vi "Create XML with many configs.vi"() -> ()   [LabVIEW 2020]
panel:
  out "Max payload size":dbl=1336.0
  out "Rx UDP Configuration":string="<?xml version=\"1.0\"?>\n<Board xmlns:xsi=\"http://www.w3.org/2001/XMLSchema-instance\" xmlns:xsd=\"http://www.w3.org/2001/XMLSchema\" BoardId=\"1\">\n  <Port PortId=\"0\">\n    <RxUdpSession VlId=\"60\" VLRange=\"1\" Bag=\"0\" Jitter=\"0\" VLBufSize=\"32768\">\n      <RxCommPort ID=\"Rx1\" DomainID=\"1\" SideID=\"1\" LocationID=\"1\" PartitionID=\"1\" UdpSrcPort=\"1\" UdpDstPort=\"1\" UdpMaxMessageSize=\"512\">\n        <Parameter>\n          <name>Param 0</name> <direction>incoming</direction> <encoding>BNR</encoding> <signed>true</signed> <startBit>0 </startBit> <numberOfBits>64</numberOfBits> <scale>1</scale> <offset>0</offset> <unit>V</unit> <defaultValue>0</defaultValue>\n        </Parameter>\n        <Parameter>\n          <name>Param 1</name> <direction>incoming</direction> <encoding>BNR</encoding> <signed>true</signed> <startBit>64 </startBit> <numberOfBits>64</numberOfBits> <scale>1</scale> <offset>0</offset> <unit>V</unit> <defaultValue>0</defaultValue>\n        </Parameter>\n        <Parameter>\n          <name>Param 2</name> <direction>incoming</direction> <encoding>BNR</encoding> <signed>true</signed> <startBit>128 </startBit> <numberOfBits>64</numberOfBits> <scale>1</scale> <offset>0</offset> <unit>V</unit> <defaultValue>0</defaultValue>\n        </Parameter>\n        <Parameter>\n          <name>Param 3</name> <direction>incoming</direction> <encoding>BNR</encoding> <signed>true</signed> <startBit>192 </startBit> <numberOfBits>64</numberOfBits> <scale>1</scale> <offset>0</offset> <unit>V</unit> <defaultValue>0</defaultValue>\n        </Parameter>\n        <Parameter>\n          <name>Param 4</name> <direction>incoming</direction> <encoding>BNR</encoding> <signed>true</signed> <startBit>256 </startBit> <numberOfBits>64</numberOfBits> <scale>1</scale> <offset>0</offset> <unit>V</unit> <defaultValue>0</defaultValue>\n        </Parameter>\n        <Parameter>\n          <name>Param 5</name> <direction>incoming</direction> <encoding>BNR</encoding> <signed>true</signed> <startBit>320 </startBit> <numberOfBits>64</numberOfBits> <scale>1</scale> <offset>0</offset> <unit>V</unit> <defaultValue>0</defaultValue>\n        </Parameter>\n        <Parameter>\n          <name>Param 6</name> <direction>incoming</direction> <encoding>BNR</encoding> <signed>true</signed> <startBit>384 </startBit> <numberOfBits>64</numberOfBits> <scale>1</scale> <offset>0</offset> <unit>V</unit> <defaultValue>0</defaultValue>\n        </Parameter>\n        <Parameter>\n          <name>Param 7</name> <direction>incoming</direction> <encoding>BNR</encoding> <signed>true</signed> <startBit>448 </startBit> <numberOfBits>64</numberOfBits> <scale>1</scale> <offset>0</offset> <unit>V</unit> <defaultValue>0</defaultValue>\n        </Parameter>\n        <Parameter>\n          <name>Param 8</name> <direction>incoming</direction> <encoding>BNR</encoding> <signed>true</signed> <startBit>512 </startBit> <numberOfBits>64</numberOfBits> <scale>1</scale> <offset>0</offset> <unit>V</unit> <defaultValue>0</defaultValue>\n        </Parameter>\n        <Parameter>\n          <name>Param 9</name> <direction>incoming</direction> <encoding>BNR</encoding> <signed>true</signed> <startBit>576 </startBit> <numberOfBits>64</numberOfBits> <scale>1</scale> <offset>0</offset> <unit>V</unit> <defaultValue>0</defaultValue>\n        </Parameter>\n        <Parameter>\n          <name>Param 10</name> <direction>incoming</direction> <encoding>BNR</encoding> <signed>true</signed> <startBit>640 </startBit> <numberOfBits>64</numberOfBits> <scale>1</scale> <offset>0</offset> <unit>V</unit> <defaultValue>0</defaultValue>\n        </Parameter>\n        <Parameter>\n          <name>Param 11</name> <direction>incoming</direction> <encoding>BNR</encoding> <signed>true</signed> <startBit>704 </startBit> <numberOfBits>64</numberOfBits> <scale>1</scale> <offset>0</offset> <unit>V</unit> <defaultValue>0</defaultValue>\n        </Parameter>\n        <Parameter>\n          <name>Param 12</name> <direction>incoming</direction> <encoding>BNR</encoding> <signed>true</signed> <startBit>768 </startBit> <numberOfBits>64</numberOfBits> <scale>1</scale> <offset>0</offset> <unit>V</unit> <defaultValue>0</defaultValue>\n        </Parameter>\n        <Parameter>\n          <name>Param 13</name> <direction>incoming</direction> <encoding>BNR</encoding> <signed>true</signed> <startBit>832 </startBit> <numberOfBits>64</numberOfBits> <scale>1</scale> <offset>0</offset> <unit>V</unit> <defaultValue>0</defaultValue>\n        </Parameter>\n        <Parameter>\n          <name>Param 14</name> <direction>incoming</direction> <encoding>BNR</encoding> <signed>true</signed> <startBit>896 </startBit> <numberOfBits>64</numberOfBits> <scale>1</scale> <offset>0</offset> <unit>V</unit> <defaultValue>0</defaultValue>\n        </Parameter>\n        <Parameter>\n          <name>Param 15</name> <direction>incoming</direction> <encoding>BNR</encoding> <signed>true</signed> <startBit>960 </startBit> <numberOfBits>64</numberOfBits> <scale>1</scale> <offset>0</offset> <unit>V</unit> <defaultValue>0</defaultValue>\n        </Parameter>\n        <Parameter>\n          <name>Param 16</name> <direction>incoming</direction> <encoding>BNR</encoding> <signed>true</signed> <startBit>1024 </startBit> <numberOfBits>64</numberOfBits> <scale>1</scale> <offset>0</offset> <unit>V</unit> <defaultValue>0</defaultValue>\n        </Parameter>\n        <Parameter>\n          <name>Param 17</name> <direction>incoming</direction> <encoding>BNR</encoding> <signed>true</signed> <startBit>1088 </startBit> <numberOfBits>64</numberOfBits> <scale>1</scale> <offset>0</offset> <unit>V</unit> <defaultValue>0</defaultValue>\n        </Parameter>\n        <Parameter>\n          <name>Param 18</name> <direction>incoming</direction> <encoding>BNR</encoding> <signed>true</signed> <startBit>1152 </startBit> <numberOfBits>64</numberOfBits> <scale>1</scale> <offset>0</offset> <unit>V</unit> <defaultValue>0</defaultValue>\n        </Parameter>\n        <Parameter>\n          <name>Param 19</name> <direction>incoming</direction> <encoding>BNR</encoding> <signed>true</signed> <startBit>1216 </startBit> <numberOfBits>64</numberOfBits> <scale>1</scale> <offset>0</offset> <unit>V</unit> <defaultValue>0</defaultValue>\n        </Parameter>\n        <Parameter>\n          <name>Param 20</name> <direction>incoming</direction> <encoding>BNR</encoding> <signed>true</signed> <startBit>1280 </startBit> <numberOfBits>64</numberOfBits> <scale>1</scale> <offset>0</offset> <unit>V</unit> <defaultValue>0</defaultValue>\n        </Parameter>\n        <Parameter>\n          <name>Param 21</name> <direction>incoming</direction> <encoding>BNR</encoding> <signed>true</signed> <startBit>1344 </startBit> <numberOfBits>64</numberOfBits> <scale>1</scale> <offset>0</offset> <unit>V</unit> <defaultValue>0</defaultValue>\n        </Parameter>\n        <Parameter>\n          <name>Param 22</name> <direction>incoming</direction> <encoding>BNR</encoding> <signed>true</signed> <startBit>1408 </startBit> <numberOfBits>64</numberOfBits> <scale>1</scale> <offset>0</offset> <unit>V</unit> <defaultValue>0</defaultValue>\n        </Parameter>\n        <Parameter>\n          <name>Param 23</name> <direction>incoming</direction> <encoding>BNR</encoding> <signed>true</signed> <startBit>1472 </startBit> <numberOfBits>64</numberOfBits> <scale>1</scale> <offset>0</offset> <unit>V</unit> <defaultValue>0</defaultValue>\n        </Parameter>\n        <Parameter>\n          <name>Param 24</name> <direction>incoming</direction> <encoding>BNR</encoding> <signed>true</signed> <startBit>1536 </startBit> <numberOfBits>64</numberOfBits> <scale>1</scale> <offset>0</offset> <unit>V</unit> <defaultValue>0</defaultValue>\n        </Parameter>\n        <Parameter>\n          <name>Param 25</name> <direction>incoming</direction> <encoding>BNR</encoding> <signed>true</signed> <startBit>1600 </startBit> <numberOfBits>64</numberOfBits> <scale>1</scale> <offset>0</offset> <unit>V</unit> <defaultValue>0</defaultValue>\n        </Parameter>\n        <Parameter>\n          <name>Param 26</name> <direction>incoming</direction> <encoding>BNR</encoding> <signed>true</signed> <startBit>1664 </startBit> <numberOfBits>64</numberOfBits> <scale>1</scale> <offset>0</offset> <unit>V</unit> <defaultValue>0</defaultValue>\n        </Parameter>\n        <Parameter>\n          <name>Param 27</name> <direction>incoming</direction> <encoding>BNR</encoding> <signed>true</signed> <startBit>1728 </startBit> <numberOfBits>64</numberOfBits> <scale>1</scale> <offset>0</offset> <unit>V</unit> <defaultValue>0</defaultValue>\n        </Parameter>\n        <Parameter>\n          <name>Param 28</name> <direction>incoming</direction> <encoding>BNR</encoding> <signed>true</signed> <startBit>1792 </startBit> <numberOfBits>64</numberOfBits> <scale>1</scale> <offset>0</offset> <unit>V</unit> <defaultValue>0</defaultValue>\n        </Parameter>\n        <Parameter>\n          <name>Param 29</name> <direction>incoming</direction> <encoding>BNR</encoding> <signed>true</signed> <startBit>1856 </startBit> <numberOfBits>64</numberOfBits> <scale>1</scale> <offset>0</offset> <unit>V</unit> <defaultValue>0</defaultValue>\n        </Parameter>\n        <Parameter>\n          <name>Param 30</name> <direction>incoming</direction> <encoding>BNR</encoding> <signed>true</signed> <startBit>1920 </startBit> <numberOfBits>64</numberOfBits> <scale>1</scale> <offset>0</offset> <unit>V</unit> <defaultValue>0</defaultValue>\n        </Parameter>\n        <Parameter>\n          <name>Param 31</name> <direction>incoming</direction> <encoding>BNR</encoding> <signed>true</signed> <startBit>1984 </startBit> <numberOfBits>64</numberOfBits> <scale>1</scale> <offset>0</offset> <unit>V</unit> <defaultValue>0</defaultValue>\n        </Parameter>\n        <Parameter>\n          <name>Param 32</name> <direction>incoming</direction> <encoding>BNR</encoding> <signed>true</signed> <startBit>2048 </startBit> <numberOfBits>64</numberOfBits> <scale>1</scale> <offset>0</offset> <unit>V</unit> <defaultValue>0</defaultValue>\n        </Parameter>\n        <Parameter>\n          <name>Param 33</name> <direction>incoming</direction> <encoding>BNR</encoding> <signed>true</signed> <startBit>2112 </startBit> <numberOfBits>64</numberOfBits> <scale>1</scale> <offset>0</offset> <unit>V</unit> <defaultValue>0</defaultValue>\n        </Parameter>\n        <Parameter>\n          <name>Param 34</name> <direction>incoming</direction> <encoding>BNR</encoding> <signed>true</signed> <startBit>2176 </startBit> <numberOfBits>64</numberOfBits> <scale>1</scale> <offset>0</offset> <unit>V</unit> <defaultValue>0</defaultValue>\n        </Parameter>\n        <Parameter>\n          <name>Param 35</name> <direction>incoming</direction> <encoding>BNR</encoding> <signed>true</signed> <startBit>2240 </startBit> <numberOfBits>64</numberOfBits> <scale>1</scale> <offset>0</offset> <unit>V</unit> <defaultValue>0</defaultValue>\n        </Parameter>\n        <Parameter>\n          <name>Param 36</name> <direction>incoming</direction> <encoding>BNR</encoding> <signed>true</signed> <startBit>2304 </startBit> <numberOfBits>64</numberOfBits> <scale>1</scale> <offset>0</offset> <unit>V</unit> <defaultValue>0</defaultValue>\n        </Parameter>\n        <Parameter>\n          <name>Param 37</name> <direction>incoming</direction> <encoding>BNR</encoding> <signed>true</signed> <startBit>2368 </startBit> <numberOfBits>64</numberOfBits> <scale>1</scale> <offset>0</offset> <unit>V</unit> <defaultValue>0</defaultValue>\n        </Parameter>\n        <Parameter>\n          <name>Param 38</name> <direction>incoming</direction> <encoding>BNR</encoding> <signed>true</signed> <startBit>2432 </startBit> <numberOfBits>64</numberOfBits> <scale>1</scale> <offset>0</offset> <unit>V</unit> <defaultValue>0</defaultValue>\n        </Parameter>\n        <Parameter>\n          <name>Param 39</name> <direction>incoming</direction> <encoding>BNR</encoding> <signed>true</signed> <startBit>2496 </startBit> <numberOfBits>64</numberOfBits> <scale>1</scale> <offset>0</offset> <unit>V</unit> <defaultValue>0</defaultValue>\n        </Parameter>\n        <Parameter>\n          <name>Param 40</name> <direction>incoming</direction> <encoding>BNR</encoding> <signed>true</signed> <startBit>2560 </startBit> <numberOfBits>64</numberOfBits> <scale>1</scale> <offset>0</offset> <unit>V</unit> <defaultValue>0</defaultValue>\n        </Parameter>\n        <Parameter>\n          <name>Param 41</name> <direction>incoming</direction> <encoding>BNR</encoding> <signed>true</signed> <startBit>2624 </startBit> <numberOfBits>64</numberOfBits> <scale>1</scale> <offset>0</offset> <unit>V</unit> <defaultValue>0</defaultValue>\n        </Parameter>\n        <Parameter>\n          <name>Param 42</name> <direction>incoming</direction> <encoding>BNR</encoding> <signed>true</signed> <startBit>2688 </startBit> <numberOfBits>64</numberOfBits> <scale>1</scale> <offset>0</offset> <unit>V</unit> <defaultValue>0</defaultValue>\n        </Parameter>\n        <Parameter>\n          <name>Param 43</name> <direction>incoming</direction> <encoding>BNR</encoding> <signed>true</signed> <startBit>2752 </startBit> <numberOfBits>64</numberOfBits> <scale>1</scale> <offset>0</offset> <unit>V</unit> <defaultValue>0</defaultValue>\n        </Parameter>\n        <Parameter>\n          <name>Param 44</name> <direction>incoming</direction> <encoding>BNR</encoding> <signed>true</signed> <startBit>2816 </startBit> <numberOfBits>64</numberOfBits> <scale>1</scale> <offset>0</offset> <unit>V</unit> <defaultValue>0</defaultValue>\n        </Parameter>\n        <Parameter>\n          <name>Param 45</name> <direction>incoming</direction> <encoding>BNR</encoding> <signed>true</signed> <startBit>2880 </startBit> <numberOfBits>64</numberOfBits> <scale>1</scale> <offset>0</offset> <unit>V</unit> <defaultValue>0</defaultValue>\n        </Parameter>\n        <Parameter>\n          <name>Param 46</name> <direction>incoming</direction> <encoding>BNR</encoding> <signed>true</signed> <startBit>2944 </startBit> <numberOfBits>64</numberOfBits> <scale>1</scale> <offset>0</offset> <unit>V</unit> <defaultValue>0</defaultValue>\n        </Parameter>\n        <Parameter>\n          <name>Param 47</name> <direction>incoming</direction> <encoding>BNR</encoding> <signed>true</signed> <startBit>3008 </startBit> <numberOfBits>64</numberOfBits> <scale>1</scale> <offset>0</offset> <unit>V</unit> <defaultValue>0</defaultValue>\n        </Parameter>\n        <Parameter>\n          <name>Param 48</name> <direction>incoming</direction> <encoding>BNR</encoding> <signed>true</signed> <startBit>3072 </startBit> <numberOfBits>64</numberOfBits> <scale>1</scale> <offset>0</offset> <unit>V</unit> <defaultValue>0</defaultValue>\n        </Parameter>\n        <Parameter>\n          <name>Param 49</name> <direction>incoming</direction> <encoding>BNR</encoding> <signed>true</signed> <startBit>3136 </startBit> <numberOfBits>64</numberOfBits> <scale>1</scale> <offset>0</offset> <unit>V</unit> <defaultValue>0</defaultValue>\n        </Parameter>\n        <Parameter>\n          <name>Param 50</name> <direction>incoming</direction> <encoding>BNR</encoding> <signed>true</signed> <startBit>3200 </startBit> <numberOfBits>64</numberOfBits> <scale>1</scale> <offset>0</offset> <unit>V</unit> <defaultValue>0</defaultValue>\n        </Parameter>\n        <Parameter>\n          <name>Param 51</name> <direction>incoming</direction> <encoding>BNR</encoding> <signed>true</signed> <startBit>3264 </startBit> <numberOfBits>64</numberOfBits> <scale>1</scale> <offset>0</offset> <unit>V</unit> <defaultValue>0</defaultValue>\n        </Parameter>\n        <Parameter>\n          <name>Param 52</name> <direction>incoming</direction> <encoding>BNR</encoding> <signed>true</signed> <startBit>3328 </startBit> <numberOfBits>64</numberOfBits> <scale>1</scale> <offset>0</offset> <unit>V</unit> <defaultValue>0</defaultValue>\n        </Parameter>\n        <Parameter>\n          <name>Param 53</name> <direction>incoming</direction> <encoding>BNR</encoding> <signed>true</signed> <startBit>3392 </startBit> <numberOfBits>64</numberOfBits> <scale>1</scale> <offset>0</offset> <unit>V</unit> <defaultValue>0</defaultValue>\n        </Parameter>\n        <Parameter>\n          <name>Param 54</name> <direction>incoming</direction> <encoding>BNR</encoding> <signed>true</signed> <startBit>3456 </startBit> <numberOfBits>64</numberOfBits> <scale>1</scale> <offset>0</offset> <unit>V</unit> <defaultValue>0</defaultValue>\n        </Parameter>\n        <Parameter>\n          <name>Param 55</name> <direction>incoming</direction> <encoding>BNR</encoding> <signed>true</signed> <startBit>3520 </startBit> <numberOfBits>64</numberOfBits> <scale>1</scale> <offset>0</offset> <unit>V</unit> <defaultValue>0</defaultValue>\n        </Parameter>\n        <Parameter>\n          <name>Param 56</name> <direction>incoming</direction> <encoding>BNR</encoding> <signed>true</signed> <startBit>3584 </startBit> <numberOfBits>64</numberOfBits> <scale>1</scale> <offset>0</offset> <unit>V</unit> <defaultValue>0</defaultValue>\n        </Parameter>\n        <Parameter>\n          <name>Param 57</name> <direction>incoming</direction> <encoding>BNR</encoding> <signed>true</signed> <startBit>3648 </startBit> <numberOfBits>64</numberOfBits> <scale>1</scale> <offset>0</offset> <unit>V</unit> <defaultValue>0</defaultValue>\n        </Parameter>\n        <Parameter>\n          <name>Param 58</name> <direction>incoming</direction> <encoding>BNR</encoding> <signed>true</signed> <startBit>3712 </startBit> <numberOfBits>64</numberOfBits> <scale>1</scale> <offset>0</offset> <unit>V</unit> <defaultValue>0</defaultValue>\n        </Parameter>\n        <Parameter>\n          <name>Param 59</name> <direction>incoming</direction> <encoding>BNR</encoding> <signed>true</signed> <startBit>3776 </startBit> <numberOfBits>64</numberOfBits> <scale>1</scale> <offset>0</offset> <unit>V</unit> <defaultValue>0</defaultValue>\n        </Parameter>\n        <Parameter>\n          <name>Param 60</name> <direction>incoming</direction> <encoding>BNR</encoding> <signed>true</signed> <startBit>3840 </startBit> <numberOfBits>64</numberOfBits> <scale>1</scale> <offset>0</offset> <unit>V</unit> <defaultValue>0</defaultValue>\n        </Parameter>\n        <Parameter>\n          <name>Param 61</name> <direction>incoming</direction> <encoding>BNR</encoding> <signed>true</signed> <startBit>3904 </startBit> <numberOfBits>64</numberOfBits> <scale>1</scale> <offset>0</offset> <unit>V</unit> <defaultValue>0</defaultValue>\n        </Parameter>\n        <Parameter>\n          <name>Param 62</name> <direction>incoming</direction> <encoding>BNR</encoding> <signed>true</signed> <startBit>3968 </startBit> <numberOfBits>64</numberOfBits> <scale>1</scale> <offset>0</offset> <unit>V</unit> <defaultValue>0</defaultValue>\n        </Parameter>\n        <Parameter>\n          <name>Param 63</name> <direction>incoming</direction> <encoding>BNR</encoding> <signed>true</signed> <startBit>4032 </startBit> <numberOfBits>64</numberOfBits> <scale>1</scale> <offset>0</offset> <unit>V</unit> <defaultValue>0</defaultValue>\n        </Parameter>\n        <Parameter>\n          <name>Param 64</name> <direction>incoming</direction> <encoding>BNR</encoding> <signed>true</signed> <startBit>4096 </startBit> <numberOfBits>64</numberOfBits> <scale>1</scale> <offset>0</offset> <unit>V</unit> <defaultValue>0</defaultValue>\n        </Parameter>\n        <Parameter>\n          <name>Param 65</name> <direction>incoming</direction> <encoding>BNR</encoding> <signed>true</signed> <startBit>4160 </startBit> <numberOfBits>64</numberOfBits> <scale>1</scale> <offset>0</offset> <unit>V</unit> <defaultValue>0</defaultValue>\n        </Parameter>\n        <Parameter>\n          <name>Param 66</name> <direction>incoming</direction> <encoding>BNR</encoding> <signed>true</signed> <startBit>4224 </startBit> <numberOfBits>64</numberOfBits> <scale>1</scale> <offset>0</offset> <unit>V</unit> <defaultValue>0</defaultValue>\n        </Parameter>\n        <Parameter>\n          <name>Param 67</name> <direction>incoming</direction> <encoding>BNR</encoding> <signed>true</signed> <startBit>4288 </startBit> <numberOfBits>64</numberOfBits> <scale>1</scale> <offset>0</offset> <unit>V</unit> <defaultValue>0</defaultValue>\n        </Parameter>\n        <Parameter>\n          <name>Param 68</name> <direction>incoming</direction> <encoding>BNR</encoding> <signed>true</signed> <startBit>4352 </startBit> <numberOfBits>64</numberOfBits> <scale>1</scale> <offset>0</offset> <unit>V</unit> <defaultValue>0</defaultValue>\n        </Parameter>\n        <Parameter>\n          <name>Param 69</name> <direction>incoming</direction> <encoding>BNR</encoding> <signed>true</signed> <startBit>4416 </startBit> <numberOfBits>64</numberOfBits> <scale>1</scale> <offset>0</offset> <unit>V</unit> <defaultValue>0</defaultValue>\n        </Parameter>\n        <Parameter>\n          <name>Param 70</name> <direction>incoming</direction> <encoding>BNR</encoding> <signed>true</signed> <startBit>4480 </startBit> <numberOfBits>64</numberOfBits> <scale>1</scale> <offset>0</offset> <unit>V</unit> <defaultValue>0</defaultValue>\n        </Parameter>\n        <Parameter>\n          <name>Param 71</name> <direction>incoming</direction> <encoding>BNR</encoding> <signed>true</signed> <startBit>4544 </startBit> <numberOfBits>64</numberOfBits> <scale>1</scale> <offset>0</offset> <unit>V</unit> <defaultValue>0</defaultValue>\n        </Parameter>\n        <Parameter>\n          <name>Param 72</name> <direction>incoming</direction> <encoding>BNR</encoding> <signed>true</signed> <startBit>4608 </startBit> <numberOfBits>64</numberOfBits> <scale>1</scale> <offset>0</offset> <unit>V</unit> <defaultValue>0</defaultValue>\n        </Parameter>\n        <Parameter>\n          <name>Param 73</name> <direction>incoming</direction> <encoding>BNR</encoding> <signed>true</signed> <startBit>4672 </startBit> <numberOfBits>64</numberOfBits> <scale>1</scale> <offset>0</offset> <unit>V</unit> <defaultValue>0</defaultValue>\n        </Parameter>\n        <Parameter>\n          <name>Param 74</name> <direction>incoming</direction> <encoding>BNR</encoding> <signed>true</signed> <startBit>4736 </startBit> <numberOfBits>64</numberOfBits> <scale>1</scale> <offset>0</offset> <unit>V</unit> <defaultValue>0</defaultValue>\n        </Parameter>\n        <Parameter>\n          <name>Param 75</name> <direction>incoming</direction> <encoding>BNR</encoding> <signed>true</signed> <startBit>4800 </startBit> <numberOfBits>64</numberOfBits> <scale>1</scale> <offset>0</offset> <unit>V</unit> <defaultValue>0</defaultValue>\n        </Parameter>\n        <Parameter>\n          <name>Param 76</name> <direction>incoming</direction> <encoding>BNR</encoding> <signed>true</signed> <startBit>4864 </startBit> <numberOfBits>64</numberOfBits> <scale>1</scale> <offset>0</offset> <unit>V</unit> <defaultValue>0</defaultValue>\n        </Parameter>\n        <Parameter>\n          <name>Param 77</name> <direction>incoming</direction> <encoding>BNR</encoding> <signed>true</signed> <startBit>4928 </startBit> <numberOfBits>64</numberOfBits> <scale>1</scale> <offset>0</offset> <unit>V</unit> <defaultValue>0</defaultValue>\n        </Parameter>\n        <Parameter>\n          <name>Param 78</name> <direction>incoming</direction> <encoding>BNR</encoding> <signed>true</signed> <startBit>4992 </startBit> <numberOfBits>64</numberOfBits> <scale>1</scale> <offset>0</offset> <unit>V</unit> <defaultValue>0</defaultValue>\n        </Parameter>\n        <Parameter>\n          <name>Param 79</name> <direction>incoming</direction> <encoding>BNR</encoding> <signed>true</signed> <startBit>5056 </startBit> <numberOfBits>64</numberOfBits> <scale>1</scale> <offset>0</offset> <unit>V</unit> <defaultValue>0</defaultValue>\n        </Parameter>\n        <Parameter>\n          <name>Param 80</name> <direction>incoming</direction> <encoding>BNR</encoding> <signed>true</signed> <startBit>5120 </startBit> <numberOfBits>64</numberOfBits> <scale>1</scale> <offset>0</offset> <unit>V</unit> <defaultValue>0</defaultValue>\n        </Parameter>\n        <Parameter>\n          <name>Param 81</name> <direction>incoming</direction> <encoding>BNR</encoding> <signed>true</signed> <startBit>5184 </startBit> <numberOfBits>64</numberOfBits> <scale>1</scale> <offset>0</offset> <unit>V</unit> <defaultValue>0</defaultValue>\n        </Parameter>\n        <Parameter>\n          <name>Param 82</name> <direction>incoming</direction> <encoding>BNR</encoding> <signed>true</signed> <startBit>5248 </startBit> <numberOfBits>64</numberOfBits> <scale>1</scale> <offset>0</offset> <unit>V</unit> <defaultValue>0</defaultValue>\n        </Parameter>\n        <Parameter>\n          <name>Param 83</name> <direction>incoming</direction> <encoding>BNR</encoding> <signed>true</signed> <startBit>5312 </startBit> <numberOfBits>64</numberOfBits> <scale>1</scale> <offset>0</offset> <unit>V</unit> <defaultValue>0</defaultValue>\n        </Parameter>\n        <Parameter>\n          <name>Param 84</name> <direction>incoming</direction> <encoding>BNR</encoding> <signed>true</signed> <startBit>5376 </startBit> <numberOfBits>64</numberOfBits> <scale>1</scale> <offset>0</offset> <unit>V</unit> <defaultValue>0</defaultValue>\n        </Parameter>\n        <Parameter>\n          <name>Param 85</name> <direction>incoming</direction> <encoding>BNR</encoding> <signed>true</signed> <startBit>5440 </startBit> <numberOfBits>64</numberOfBits> <scale>1</scale> <offset>0</offset> <unit>V</unit> <defaultValue>0</defaultValue>\n        </Parameter>\n        <Parameter>\n          <name>Param 86</name> <direction>incoming</direction> <encoding>BNR</encoding> <signed>true</signed> <startBit>5504 </startBit> <numberOfBits>64</numberOfBits> <scale>1</scale> <offset>0</offset> <unit>V</unit> <defaultValue>0</defaultValue>\n        </Parameter>\n        <Parameter>\n          <name>Param 87</name> <direction>incoming</direction> <encoding>BNR</encoding> <signed>true</signed> <startBit>5568 </startBit> <numberOfBits>64</numberOfBits> <scale>1</scale> <offset>0</offset> <unit>V</unit> <defaultValue>0</defaultValue>\n        </Parameter>\n        <Parameter>\n          <name>Param 88</name> <direction>incoming</direction> <encoding>BNR</encoding> <signed>true</signed> <startBit>5632 </startBit> <numberOfBits>64</numberOfBits> <scale>1</scale> <offset>0</offset> <unit>V</unit> <defaultValue>0</defaultValue>\n        </Parameter>\n        <Parameter>\n          <name>Param 89</name> <direction>incoming</direction> <encoding>BNR</encoding> <signed>true</signed> <startBit>5696 </startBit> <numberOfBits>64</numberOfBits> <scale>1</scale> <offset>0</offset> <unit>V</unit> <defaultValue>0</defaultValue>\n        </Parameter>\n        <Parameter>\n          <name>Param 90</name> <direction>incoming</direction> <encoding>BNR</encoding> <signed>true</signed> <startBit>5760 </startBit> <numberOfBits>64</numberOfBits> <scale>1</scale> <offset>0</offset> <unit>V</unit> <defaultValue>0</defaultValue>\n        </Parameter>\n        <Parameter>\n          <name>Param 91</name> <direction>incoming</direction> <encoding>BNR</encoding> <signed>true</signed> <startBit>5824 </startBit> <numberOfBits>64</numberOfBits> <scale>1</scale> <offset>0</offset> <unit>V</unit> <defaultValue>0</defaultValue>\n        </Parameter>\n        <Parameter>\n          <name>Param 92</name> <direction>incoming</direction> <encoding>BNR</encoding> <signed>true</signed> <startBit>5888 </startBit> <numberOfBits>64</numberOfBits> <scale>1</scale> <offset>0</offset> <unit>V</unit> <defaultValue>0</defaultValue>\n        </Parameter>\n        <Parameter>\n          <name>Param 93</name> <direction>incoming</direction> <encoding>BNR</encoding> <signed>true</signed> <startBit>5952 </startBit> <numberOfBits>64</numberOfBits> <scale>1</scale> <offset>0</offset> <unit>V</unit> <defaultValue>0</defaultValue>\n        </Parameter>\n        <Parameter>\n          <name>Param 94</name> <direction>incoming</direction> <encoding>BNR</encoding> <signed>true</signed> <startBit>6016 </startBit> <numberOfBits>64</numberOfBits> <scale>1</scale> <offset>0</offset> <unit>V</unit> <defaultValue>0</defaultValue>\n        </Parameter>\n        <Parameter>\n          <name>Param 95</name> <direction>incoming</direction> <encoding>BNR</encoding> <signed>true</signed> <startBit>6080 </startBit> <numberOfBits>64</numberOfBits> <scale>1</scale> <offset>0</offset> <unit>V</unit> <defaultValue>0</defaultValue>\n        </Parameter>\n        <Parameter>\n          <name>Param 96</name> <direction>incoming</direction> <encoding>BNR</encoding> <signed>true</signed> <startBit>6144 </startBit> <numberOfBits>64</numberOfBits> <scale>1</scale> <offset>0</offset> <unit>V</unit> <defaultValue>0</defaultValue>\n        </Parameter>\n        <Parameter>\n          <name>Param 97</name> <direction>incoming</direction> <encoding>BNR</encoding> <signed>true</signed> <startBit>6208 </startBit> <numberOfBits>64</numberOfBits> <scale>1</scale> <offset>0</offset> <unit>V</unit> <defaultValue>0</defaultValue>\n        </Parameter>\n        <Parameter>\n          <name>Param 98</name> <direction>incoming</direction> <encoding>BNR</encoding> <signed>true</signed> <startBit>6272 </startBit> <numberOfBits>64</numberOfBits> <scale>1</scale> <offset>0</offset> <unit>V</unit> <defaultValue>0</defaultValue>\n        </Parameter>\n        <Parameter>\n          <name>Param 99</name> <direction>incoming</direction> <encoding>BNR</encoding> <signed>true</signed> <startBit>6336 </startBit> <numberOfBits>64</numberOfBits> <scale>1</scale> <offset>0</offset> <unit>V</unit> <defaultValue>0</defaultValue>\n        </Parameter>\n        <Parameter>\n          <name>Param 100</name> <direction>incoming</direction> <encoding>BNR</encoding> <signed>true</signed> <startBit>6400 </startBit> <numberOfBits>64</numberOfBits> <scale>1</scale> <offset>0</offset> <unit>V</unit> <defaultValue>0</defaultValue>\n        </Parameter>\n        <Parameter>\n          <name>Param 101</name> <direction>incoming</direction> <encoding>BNR</encoding> <signed>true</signed> <startBit>6464 </startBit> <numberOfBits>64</numberOfBits> <scale>1</scale> <offset>0</offset> <unit>V</unit> <defaultValue>0</defaultValue>\n        </Parameter>\n        <Parameter>\n          <name>Param 102</name> <direction>incoming</direction> <encoding>BNR</encoding> <signed>true</signed> <startBit>6528 </startBit> <numberOfBits>64</numberOfBits> <scale>1</scale> <offset>0</offset> <unit>V</unit> <defaultValue>0</defaultValue>\n        </Parameter>\n        <Parameter>\n          <name>Param 103</name> <direction>incoming</direction> <encoding>BNR</encoding> <signed>true</signed> <startBit>6592 </startBit> <numberOfBits>64</numberOfBits> <scale>1</scale> <offset>0</offset> <unit>V</unit> <defaultValue>0</defaultValue>\n        </Parameter>\n        <Parameter>\n          <name>Param 104</name> <direction>incoming</direction> <encoding>BNR</encoding> <signed>true</signed> <startBit>6656 </startBit> <numberOfBits>64</numberOfBits> <scale>1</scale> <offset>0</offset> <unit>V</unit> <defaultValue>0</defaultValue>\n        </Parameter>\n        <Parameter>\n          <name>Param 105</name> <direction>incoming</direction> <encoding>BNR</encoding> <signed>true</signed> <startBit>6720 </startBit> <numberOfBits>64</numberOfBits> <scale>1</scale> <offset>0</offset> <unit>V</unit> <defaultValue>0</defaultValue>\n        </Parameter>\n        <Parameter>\n          <name>Param 106</name> <direction>incoming</direction> <encoding>BNR</encoding> <signed>true</signed> <startBit>6784 </startBit> <numberOfBits>64</numberOfBits> <scale>1</scale> <offset>0</offset> <unit>V</unit> <defaultValue>0</defaultValue>\n        </Parameter>\n        <Parameter>\n          <name>Param 107</name> <direction>incoming</direction> <encoding>BNR</encoding> <signed>true</signed> <startBit>6848 </startBit> <numberOfBits>64</numberOfBits> <scale>1</scale> <offset>0</offset> <unit>V</unit> <defaultValue>0</defaultValue>\n        </Parameter>\n        <Parameter>\n          <name>Param 108</name> <direction>incoming</direction> <encoding>BNR</encoding> <signed>true</signed> <startBit>6912 </startBit> <numberOfBits>64</numberOfBits> <scale>1</scale> <offset>0</offset> <unit>V</unit> <defaultValue>0</defaultValue>\n        </Parameter>\n        <Parameter>\n          <name>Param 109</name> <direction>incoming</direction> <encoding>BNR</encoding> <signed>true</signed> <startBit>6976 </startBit> <numberOfBits>64</numberOfBits> <scale>1</scale> <offset>0</offset> <unit>V</unit> <defaultValue>0</defaultValue>\n        </Parameter>\n        <Parameter>\n          <name>Param 110</name> <direction>incoming</direction> <encoding>BNR</encoding> <signed>true</signed> <startBit>7040 </startBit> <numberOfBits>64</numberOfBits> <scale>1</scale> <offset>0</offset> <unit>V</unit> <defaultValue>0</defaultValue>\n        </Parameter>\n        <Parameter>\n          <name>Param 111</name> <direction>incoming</direction> <encoding>BNR</encoding> <signed>true</signed> <startBit>7104 </startBit> <numberOfBits>64</numberOfBits> <scale>1</scale> <offset>0</offset> <unit>V</unit> <defaultValue>0</defaultValue>\n        </Parameter>\n        <Parameter>\n          <name>Param 112</name> <direction>incoming</direction> <encoding>BNR</encoding> <signed>true</signed> <startBit>7168 </startBit> <numberOfBits>64</numberOfBits> <scale>1</scale> <offset>0</offset> <unit>V</unit> <defaultValue>0</defaultValue>\n        </Parameter>\n        <Parameter>\n          <name>Param 113</name> <direction>incoming</direction> <encoding>BNR</encoding> <signed>true</signed> <startBit>7232 </startBit> <numberOfBits>64</numberOfBits> <scale>1</scale> <offset>0</offset> <unit>V</unit> <defaultValue>0</defaultValue>\n        </Parameter>\n        <Parameter>\n          <name>Param 114</name> <direction>incoming</direction> <encoding>BNR</encoding> <signed>true</signed> <startBit>7296 </startBit> <numberOfBits>64</numberOfBits> <scale>1</scale> <offset>0</offset> <unit>V</unit> <defaultValue>0</defaultValue>\n        </Parameter>\n        <Parameter>\n          <name>Param 115</name> <direction>incoming</direction> <encoding>BNR</encoding> <signed>true</signed> <startBit>7360 </startBit> <numberOfBits>64</numberOfBits> <scale>1</scale> <offset>0</offset> <unit>V</unit> <defaultValue>0</defaultValue>\n        </Parameter>\n        <Parameter>\n          <name>Param 116</name> <direction>incoming</direction> <encoding>BNR</encoding> <signed>true</signed> <startBit>7424 </startBit> <numberOfBits>64</numberOfBits> <scale>1</scale> <offset>0</offset> <unit>V</unit> <defaultValue>0</defaultValue>\n        </Parameter>\n        <Parameter>\n          <name>Param 117</name> <direction>incoming</direction> <encoding>BNR</encoding> <signed>true</signed> <startBit>7488 </startBit> <numberOfBits>64</numberOfBits> <scale>1</scale> <offset>0</offset> <unit>V</unit> <defaultValue>0</defaultValue>\n        </Parameter>\n        <Parameter>\n          <name>Param 118</name> <direction>incoming</direction> <encoding>BNR</encoding> <signed>true</signed> <startBit>7552 </startBit> <numberOfBits>64</numberOfBits> <scale>1</scale> <offset>0</offset> <unit>V</unit> <defaultValue>0</defaultValue>\n        </Parameter>\n        <Parameter>\n          <name>Param 119</name> <direction>incoming</direction> <encoding>BNR</encoding> <signed>true</signed> <startBit>7616 </startBit> <numberOfBits>64</numberOfBits> <scale>1</scale> <offset>0</offset> <unit>V</unit> <defaultValue>0</defaultValue>\n        </Parameter>\n        <Parameter>\n          <name>Param 120</name> <direction>incoming</direction> <encoding>BNR</encoding> <signed>true</signed> <startBit>7680 </startBit> <numberOfBits>64</numberOfBits> <scale>1</scale> <offset>0</offset> <unit>V</unit> <defaultValue>0</defaultValue>\n        </Parameter>\n        <Parameter>\n          <name>Param 121</name> <direction>incoming</direction> <encoding>BNR</encoding> <signed>true</signed> <startBit>7744 </startBit> <numberOfBits>64</numberOfBits> <scale>1</scale> <offset>0</offset> <unit>V</unit> <defaultValue>0</defaultValue>\n        </Parameter>\n        <Parameter>\n          <name>Param 122</name> <direction>incoming</direction> <encoding>BNR</encoding> <signed>true</signed> <startBit>7808 </startBit> <numberOfBits>64</numberOfBits> <scale>1</scale> <offset>0</offset> <unit>V</unit> <defaultValue>0</defaultValue>\n        </Parameter>\n        <Parameter>\n          <name>Param 123</name> <direction>incoming</direction> <encoding>BNR</encoding> <signed>true</signed> <startBit>7872 </startBit> <numberOfBits>64</numberOfBits> <scale>1</scale> <offset>0</offset> <unit>V</unit> <defaultValue>0</defaultValue>\n        </Parameter>\n        <Parameter>\n          <name>Param 124</name> <direction>incoming</direction> <encoding>BNR</encoding> <signed>true</signed> <startBit>7936 </startBit> <numberOfBits>64</numberOfBits> <scale>1</scale> <offset>0</offset> <unit>V</unit> <defaultValue>0</defaultValue>\n        </Parameter>\n        <Parameter>\n          <name>Param 125</name> <direction>incoming</direction> <encoding>BNR</encoding> <signed>true</signed> <startBit>8000 </startBit> <numberOfBits>64</numberOfBits> <scale>1</scale> <offset>0</offset> <unit>V</unit> <defaultValue>0</defaultValue>\n        </Parameter>\n        <Parameter>\n          <name>Param 126</name> <direction>incoming</direction> <encoding>BNR</encoding> <signed>true</signed> <startBit>8064 </startBit> <numberOfBits>64</numberOfBits> <scale>1</scale> <offset>0</offset> <unit>V</unit> <defaultValue>0</defaultValue>\n        </Parameter>\n        <Parameter>\n          <name>Param 127</name> <direction>incoming</direction> <encoding>BNR</encoding> <signed>true</signed> <startBit>8128 </startBit> <numberOfBits>64</numberOfBits> <scale>1</scale> <offset>0</offset> <unit>V</unit> <defaultValue>0</defaultValue>\n        </Parameter>\n        <Parameter>\n          <name>Param 128</name> <direction>incoming</direction> <encoding>BNR</encoding> <signed>true</signed> <startBit>8192 </startBit> <numberOfBits>64</numberOfBits> <scale>1</scale> <offset>0</offset> <unit>V</unit> <defaultValue>0</defaultValue>\n        </Parameter>\n        <Parameter>\n          <name>Param 129</name> <direction>incoming</direction> <encoding>BNR</encoding> <signed>true</signed> <startBit>8256 </startBit> <numberOfBits>64</numberOfBits> <scale>1</scale> <offset>0</offset> <unit>V</unit> <defaultValue>0</defaultValue>\n        </Parameter>\n        <Parameter>\n          <name>Param 130</name> <direction>incoming</direction> <encoding>BNR</encoding> <signed>true</signed> <startBit>8320 </startBit> <numberOfBits>64</numberOfBits> <scale>1</scale> <offset>0</offset> <unit>V</unit> <defaultValue>0</defaultValue>\n        </Parameter>\n        <Parameter>\n          <name>Param 131</name> <direction>incoming</direction> <encoding>BNR</encoding> <signed>true</signed> <startBit>8384 </startBit> <numberOfBits>64</numberOfBits> <scale>1</scale> <offset>0</offset> <unit>V</unit> <defaultValue>0</defaultValue>\n        </Parameter>\n        <Parameter>\n          <name>Param 132</name> <direction>incoming</direction> <encoding>BNR</encoding> <signed>true</signed> <startBit>8448 </startBit> <numberOfBits>64</numberOfBits> <scale>1</scale> <offset>0</offset> <unit>V</unit> <defaultValue>0</defaultValue>\n        </Parameter>\n        <Parameter>\n          <name>Param 133</name> <direction>incoming</direction> <encoding>BNR</encoding> <signed>true</signed> <startBit>8512 </startBit> <numberOfBits>64</numberOfBits> <scale>1</scale> <offset>0</offset> <unit>V</unit> <defaultValue>0</defaultValue>\n        </Parameter>\n        <Parameter>\n          <name>Param 134</name> <direction>incoming</direction> <encoding>BNR</encoding> <signed>true</signed> <startBit>8576 </startBit> <numberOfBits>64</numberOfBits> <scale>1</scale> <offset>0</offset> <unit>V</unit> <defaultValue>0</defaultValue>\n        </Parameter>\n        <Parameter>\n          <name>Param 135</name> <direction>incoming</direction> <encoding>BNR</encoding> <signed>true</signed> <startBit>8640 </startBit> <numberOfBits>64</numberOfBits> <scale>1</scale> <offset>0</offset> <unit>V</unit> <defaultValue>0</defaultValue>\n        </Parameter>\n        <Parameter>\n          <name>Param 136</name> <direction>incoming</direction> <encoding>BNR</encoding> <signed>true</signed> <startBit>8704 </startBit> <numberOfBits>64</numberOfBits> <scale>1</scale> <offset>0</offset> <unit>V</unit> <defaultValue>0</defaultValue>\n        </Parameter>\n        <Parameter>\n          <name>Param 137</name> <direction>incoming</direction> <encoding>BNR</encoding> <signed>true</signed> <startBit>8768 </startBit> <numberOfBits>64</numberOfBits> <scale>1</scale> <offset>0</offset> <unit>V</unit> <defaultValue>0</defaultValue>\n        </Parameter>\n        <Parameter>\n          <name>Param 138</name> <direction>incoming</direction> <encoding>BNR</encoding> <signed>true</signed> <startBit>8832 </startBit> <numberOfBits>64</numberOfBits> <scale>1</scale> <offset>0</offset> <unit>V</unit> <defaultValue>0</defaultValue>\n        </Parameter>\n        <Parameter>\n          <name>Param 139</name> <direction>incoming</direction> <encoding>BNR</encoding> <signed>true</signed> <startBit>8896 </startBit> <numberOfBits>64</numberOfBits> <scale>1</scale> <offset>0</offset> <unit>V</unit> <defaultValue>0</defaultValue>\n        </Parameter>\n        <Parameter>\n          <name>Param 140</name> <direction>incoming</direction> <encoding>BNR</encoding> <signed>true</signed> <startBit>8960 </startBit> <numberOfBits>64</numberOfBits> <scale>1</scale> <offset>0</offset> <unit>V</unit> <defaultValue>0</defaultValue>\n        </Parameter>\n        <Parameter>\n          <name>Param 141</name> <direction>incoming</direction> <encoding>BNR</encoding> <signed>true</signed> <startBit>9024 </startBit> <numberOfBits>64</numberOfBits> <scale>1</scale> <offset>0</offset> <unit>V</unit> <defaultValue>0</defaultValue>\n        </Parameter>\n        <Parameter>\n          <name>Param 142</name> <direction>incoming</direction> <encoding>BNR</encoding> <signed>true</signed> <startBit>9088 </startBit> <numberOfBits>64</numberOfBits> <scale>1</scale> <offset>0</offset> <unit>V</unit> <defaultValue>0</defaultValue>\n        </Parameter>\n        <Parameter>\n          <name>Param 143</name> <direction>incoming</direction> <encoding>BNR</encoding> <signed>true</signed> <startBit>9152 </startBit> <numberOfBits>64</numberOfBits> <scale>1</scale> <offset>0</offset> <unit>V</unit> <defaultValue>0</defaultValue>\n        </Parameter>\n        <Parameter>\n          <name>Param 144</name> <direction>incoming</direction> <encoding>BNR</encoding> <signed>true</signed> <startBit>9216 </startBit> <numberOfBits>64</numberOfBits> <scale>1</scale> <offset>0</offset> <unit>V</unit> <defaultValue>0</defaultValue>\n        </Parameter>\n        <Parameter>\n          <name>Param 145</name> <direction>incoming</direction> <encoding>BNR</encoding> <signed>true</signed> <startBit>9280 </startBit> <numberOfBits>64</numberOfBits> <scale>1</scale> <offset>0</offset> <unit>V</unit> <defaultValue>0</defaultValue>\n        </Parameter>\n        <Parameter>\n          <name>Param 146</name> <direction>incoming</direction> <encoding>BNR</encoding> <signed>true</signed> <startBit>9344 </startBit> <numberOfBits>64</numberOfBits> <scale>1</scale> <offset>0</offset> <unit>V</unit> <defaultValue>0</defaultValue>\n        </Parameter>\n        <Parameter>\n          <name>Param 147</name> <direction>incoming</direction> <encoding>BNR</encoding> <signed>true</signed> <startBit>9408 </startBit> <numberOfBits>64</numberOfBits> <scale>1</scale> <offset>0</offset> <unit>V</unit> <defaultValue>0</defaultValue>\n        </Parameter>\n        <Parameter>\n          <name>Param 148</name> <direction>incoming</direction> <encoding>BNR</encoding> <signed>true</signed> <startBit>9472 </startBit> <numberOfBits>64</numberOfBits> <scale>1</scale> <offset>0</offset> <unit>V</unit> <defaultValue>0</defaultValue>\n        </Parameter>\n        <Parameter>\n          <name>Param 149</name> <direction>incoming</direction> <encoding>BNR</encoding> <signed>true</signed> <startBit>9536 </startBit> <numberOfBits>64</numberOfBits> <scale>1</scale> <offset>0</offset> <unit>V</unit> <defaultValue>0</defaultValue>\n        </Parameter>\n        <Parameter>\n          <name>Param 150</name> <direction>incoming</direction> <encoding>BNR</encoding> <signed>true</signed> <startBit>9600 </startBit> <numberOfBits>64</numberOfBits> <scale>1</scale> <offset>0</offset> <unit>V</unit> <defaultValue>0</defaultValue>\n        </Parameter>\n        <Parameter>\n          <name>Param 151</name> <direction>incoming</direction> <encoding>BNR</encoding> <signed>true</signed> <startBit>9664 </startBit> <numberOfBits>64</numberOfBits> <scale>1</scale> <offset>0</offset> <unit>V</unit> <defaultValue>0</defaultValue>\n        </Parameter>\n        <Parameter>\n          <name>Param 152</name> <direction>incoming</direction> <encoding>BNR</encoding> <signed>true</signed> <startBit>9728 </startBit> <numberOfBits>64</numberOfBits> <scale>1</scale> <offset>0</offset> <unit>V</unit> <defaultValue>0</defaultValue>\n        </Parameter>\n        <Parameter>\n          <name>Param 153</name> <direction>incoming</direction> <encoding>BNR</encoding> <signed>true</signed> <startBit>9792 </startBit> <numberOfBits>64</numberOfBits> <scale>1</scale> <offset>0</offset> <unit>V</unit> <defaultValue>0</defaultValue>\n        </Parameter>\n        <Parameter>\n          <name>Param 154</name> <direction>incoming</direction> <encoding>BNR</encoding> <signed>true</signed> <startBit>9856 </startBit> <numberOfBits>64</numberOfBits> <scale>1</scale> <offset>0</offset> <unit>V</unit> <defaultValue>0</defaultValue>\n        </Parameter>\n        <Parameter>\n          <name>Param 155</name> <direction>incoming</direction> <encoding>BNR</encoding> <signed>true</signed> <startBit>9920 </startBit> <numberOfBits>64</numberOfBits> <scale>1</scale> <offset>0</offset> <unit>V</unit> <defaultValue>0</defaultValue>\n        </Parameter>\n        <Parameter>\n          <name>Param 156</name> <direction>incoming</direction> <encoding>BNR</encoding> <signed>true</signed> <startBit>9984 </startBit> <numberOfBits>64</numberOfBits> <scale>1</scale> <offset>0</offset> <unit>V</unit> <defaultValue>0</defaultValue>\n        </Parameter>\n        <Parameter>\n          <name>Param 157</name> <direction>incoming</direction> <encoding>BNR</encoding> <signed>true</signed> <startBit>10048 </startBit> <numberOfBits>64</numberOfBits> <scale>1</scale> <offset>0</offset> <unit>V</unit> <defaultValue>0</defaultValue>\n        </Parameter>\n        <Parameter>\n          <name>Param 158</name> <direction>incoming</direction> <encoding>BNR</encoding> <signed>true</signed> <startBit>10112 </startBit> <numberOfBits>64</numberOfBits> <scale>1</scale> <offset>0</offset> <unit>V</unit> <defaultValue>0</defaultValue>\n        </Parameter>\n        <Parameter>\n          <name>Param 159</name> <direction>incoming</direction> <encoding>BNR</encoding> <signed>true</signed> <startBit>10176 </startBit> <numberOfBits>64</numberOfBits> <scale>1</scale> <offset>0</offset> <unit>V</unit> <defaultValue>0</defaultValue>\n        </Parameter>\n      </RxCommPort>\n    </RxUdpSession>\n  </Port>\n</Board>"
  in  "Rx with N Parameters":path=path "D:/git/niveristand-aim-arinc664-custom-device/Source/Custom Device Support/Tests/System/AIM ARINC 664 Loopback/Assets/UDP_RX_TX_Loopback-Board 1-Parameters 160- 1 UDP Port.xml"
  in  "Numeric":i32=160
  in  "Tx with N Parameters":path=path "D:/git/niveristand-aim-arinc664-custom-device/Source/Custom Device Support/Tests/System/AIM ARINC 664 Loopback/Assets/UDP_RX_TX_Loopback-Board 0-Parameters 160- 1 UDP Port.xml"
  out "Tx UDP Configuration":string="<?xml version=\"1.0\"?>\n<Board xmlns:xsi=\"http://www.w3.org/2001/XMLSchema-instance\" xmlns:xsd=\"http://www.w3.org/2001/XMLSchema\">\n  <Port PortId=\"0\">\n    <TxUdpSession VlId=\"60\" Bag=\"64\" DomainID=\"1\" SideID=\"1\" LocationID=\"1\" InterfaceID=\"1\" MaxFrameLength=\"1518\">\n      <TxCommPort ID=\"Tx1\" PartitionID=\"1\" UdpSrcPort=\"1\" UdpDstPort=\"1\" UdpSamplingRate=\"64\" UdpMaxMessageSize=\"512\">\n        <Parameter>\n          <name>Param 0</name> <direction>outgoing</direction> <encoding>BNR</encoding> <signed>true</signed> <startBit>0 </startBit> <numberOfBits>64</numberOfBits> <scale>1</scale> <offset>0</offset> <unit>V</unit> <defaultValue>0</defaultValue>\n        </Parameter>\n        <Parameter>\n          <name>Param 1</name> <direction>outgoing</direction> <encoding>BNR</encoding> <signed>true</signed> <startBit>64 </startBit> <numberOfBits>64</numberOfBits> <scale>1</scale> <offset>0</offset> <unit>V</unit> <defaultValue>0</defaultValue>\n        </Parameter>\n        <Parameter>\n          <name>Param 2</name> <direction>outgoing</direction> <encoding>BNR</encoding> <signed>true</signed> <startBit>128 </startBit> <numberOfBits>64</numberOfBits> <scale>1</scale> <offset>0</offset> <unit>V</unit> <defaultValue>0</defaultValue>\n        </Parameter>\n        <Parameter>\n          <name>Param 3</name> <direction>outgoing</direction> <encoding>BNR</encoding> <signed>true</signed> <startBit>192 </startBit> <numberOfBits>64</numberOfBits> <scale>1</scale> <offset>0</offset> <unit>V</unit> <defaultValue>0</defaultValue>\n        </Parameter>\n        <Parameter>\n          <name>Param 4</name> <direction>outgoing</direction> <encoding>BNR</encoding> <signed>true</signed> <startBit>256 </startBit> <numberOfBits>64</numberOfBits> <scale>1</scale> <offset>0</offset> <unit>V</unit> <defaultValue>0</defaultValue>\n        </Parameter>\n        <Parameter>\n          <name>Param 5</name> <direction>outgoing</direction> <encoding>BNR</encoding> <signed>true</signed> <startBit>320 </startBit> <numberOfBits>64</numberOfBits> <scale>1</scale> <offset>0</offset> <unit>V</unit> <defaultValue>0</defaultValue>\n        </Parameter>\n        <Parameter>\n          <name>Param 6</name> <direction>outgoing</direction> <encoding>BNR</encoding> <signed>true</signed> <startBit>384 </startBit> <numberOfBits>64</numberOfBits> <scale>1</scale> <offset>0</offset> <unit>V</unit> <defaultValue>0</defaultValue>\n        </Parameter>\n        <Parameter>\n          <name>Param 7</name> <direction>outgoing</direction> <encoding>BNR</encoding> <signed>true</signed> <startBit>448 </startBit> <numberOfBits>64</numberOfBits> <scale>1</scale> <offset>0</offset> <unit>V</unit> <defaultValue>0</defaultValue>\n        </Parameter>\n        <Parameter>\n          <name>Param 8</name> <direction>outgoing</direction> <encoding>BNR</encoding> <signed>true</signed> <startBit>512 </startBit> <numberOfBits>64</numberOfBits> <scale>1</scale> <offset>0</offset> <unit>V</unit> <defaultValue>0</defaultValue>\n        </Parameter>\n        <Parameter>\n          <name>Param 9</name> <direction>outgoing</direction> <encoding>BNR</encoding> <signed>true</signed> <startBit>576 </startBit> <numberOfBits>64</numberOfBits> <scale>1</scale> <offset>0</offset> <unit>V</unit> <defaultValue>0</defaultValue>\n        </Parameter>\n        <Parameter>\n          <name>Param 10</name> <direction>outgoing</direction> <encoding>BNR</encoding> <signed>true</signed> <startBit>640 </startBit> <numberOfBits>64</numberOfBits> <scale>1</scale> <offset>0</offset> <unit>V</unit> <defaultValue>0</defaultValue>\n        </Parameter>\n        <Parameter>\n          <name>Param 11</name> <direction>outgoing</direction> <encoding>BNR</encoding> <signed>true</signed> <startBit>704 </startBit> <numberOfBits>64</numberOfBits> <scale>1</scale> <offset>0</offset> <unit>V</unit> <defaultValue>0</defaultValue>\n        </Parameter>\n        <Parameter>\n          <name>Param 12</name> <direction>outgoing</direction> <encoding>BNR</encoding> <signed>true</signed> <startBit>768 </startBit> <numberOfBits>64</numberOfBits> <scale>1</scale> <offset>0</offset> <unit>V</unit> <defaultValue>0</defaultValue>\n        </Parameter>\n        <Parameter>\n          <name>Param 13</name> <direction>outgoing</direction> <encoding>BNR</encoding> <signed>true</signed> <startBit>832 </startBit> <numberOfBits>64</numberOfBits> <scale>1</scale> <offset>0</offset> <unit>V</unit> <defaultValue>0</defaultValue>\n        </Parameter>\n        <Parameter>\n          <name>Param 14</name> <direction>outgoing</direction> <encoding>BNR</encoding> <signed>true</signed> <startBit>896 </startBit> <numberOfBits>64</numberOfBits> <scale>1</scale> <offset>0</offset> <unit>V</unit> <defaultValue>0</defaultValue>\n        </Parameter>\n        <Parameter>\n          <name>Param 15</name> <direction>outgoing</direction> <encoding>BNR</encoding> <signed>true</signed> <startBit>960 </startBit> <numberOfBits>64</numberOfBits> <scale>1</scale> <offset>0</offset> <unit>V</unit> <defaultValue>0</defaultValue>\n        </Parameter>\n        <Parameter>\n          <name>Param 16</name> <direction>outgoing</direction> <encoding>BNR</encoding> <signed>true</signed> <startBit>1024 </startBit> <numberOfBits>64</numberOfBits> <scale>1</scale> <offset>0</offset> <unit>V</unit> <defaultValue>0</defaultValue>\n        </Parameter>\n        <Parameter>\n          <name>Param 17</name> <direction>outgoing</direction> <encoding>BNR</encoding> <signed>true</signed> <startBit>1088 </startBit> <numberOfBits>64</numberOfBits> <scale>1</scale> <offset>0</offset> <unit>V</unit> <defaultValue>0</defaultValue>\n        </Parameter>\n        <Parameter>\n          <name>Param 18</name> <direction>outgoing</direction> <encoding>BNR</encoding> <signed>true</signed> <startBit>1152 </startBit> <numberOfBits>64</numberOfBits> <scale>1</scale> <offset>0</offset> <unit>V</unit> <defaultValue>0</defaultValue>\n        </Parameter>\n        <Parameter>\n          <name>Param 19</name> <direction>outgoing</direction> <encoding>BNR</encoding> <signed>true</signed> <startBit>1216 </startBit> <numberOfBits>64</numberOfBits> <scale>1</scale> <offset>0</offset> <unit>V</unit> <defaultValue>0</defaultValue>\n        </Parameter>\n        <Parameter>\n          <name>Param 20</name> <direction>outgoing</direction> <encoding>BNR</encoding> <signed>true</signed> <startBit>1280 </startBit> <numberOfBits>64</numberOfBits> <scale>1</scale> <offset>0</offset> <unit>V</unit> <defaultValue>0</defaultValue>\n        </Parameter>\n        <Parameter>\n          <name>Param 21</name> <direction>outgoing</direction> <encoding>BNR</encoding> <signed>true</signed> <startBit>1344 </startBit> <numberOfBits>64</numberOfBits> <scale>1</scale> <offset>0</offset> <unit>V</unit> <defaultValue>0</defaultValue>\n        </Parameter>\n        <Parameter>\n          <name>Param 22</name> <direction>outgoing</direction> <encoding>BNR</encoding> <signed>true</signed> <startBit>1408 </startBit> <numberOfBits>64</numberOfBits> <scale>1</scale> <offset>0</offset> <unit>V</unit> <defaultValue>0</defaultValue>\n        </Parameter>\n        <Parameter>\n          <name>Param 23</name> <direction>outgoing</direction> <encoding>BNR</encoding> <signed>true</signed> <startBit>1472 </startBit> <numberOfBits>64</numberOfBits> <scale>1</scale> <offset>0</offset> <unit>V</unit> <defaultValue>0</defaultValue>\n        </Parameter>\n        <Parameter>\n          <name>Param 24</name> <direction>outgoing</direction> <encoding>BNR</encoding> <signed>true</signed> <startBit>1536 </startBit> <numberOfBits>64</numberOfBits> <scale>1</scale> <offset>0</offset> <unit>V</unit> <defaultValue>0</defaultValue>\n        </Parameter>\n        <Parameter>\n          <name>Param 25</name> <direction>outgoing</direction> <encoding>BNR</encoding> <signed>true</signed> <startBit>1600 </startBit> <numberOfBits>64</numberOfBits> <scale>1</scale> <offset>0</offset> <unit>V</unit> <defaultValue>0</defaultValue>\n        </Parameter>\n        <Parameter>\n          <name>Param 26</name> <direction>outgoing</direction> <encoding>BNR</encoding> <signed>true</signed> <startBit>1664 </startBit> <numberOfBits>64</numberOfBits> <scale>1</scale> <offset>0</offset> <unit>V</unit> <defaultValue>0</defaultValue>\n        </Parameter>\n        <Parameter>\n          <name>Param 27</name> <direction>outgoing</direction> <encoding>BNR</encoding> <signed>true</signed> <startBit>1728 </startBit> <numberOfBits>64</numberOfBits> <scale>1</scale> <offset>0</offset> <unit>V</unit> <defaultValue>0</defaultValue>\n        </Parameter>\n        <Parameter>\n          <name>Param 28</name> <direction>outgoing</direction> <encoding>BNR</encoding> <signed>true</signed> <startBit>1792 </startBit> <numberOfBits>64</numberOfBits> <scale>1</scale> <offset>0</offset> <unit>V</unit> <defaultValue>0</defaultValue>\n        </Parameter>\n        <Parameter>\n          <name>Param 29</name> <direction>outgoing</direction> <encoding>BNR</encoding> <signed>true</signed> <startBit>1856 </startBit> <numberOfBits>64</numberOfBits> <scale>1</scale> <offset>0</offset> <unit>V</unit> <defaultValue>0</defaultValue>\n        </Parameter>\n        <Parameter>\n          <name>Param 30</name> <direction>outgoing</direction> <encoding>BNR</encoding> <signed>true</signed> <startBit>1920 </startBit> <numberOfBits>64</numberOfBits> <scale>1</scale> <offset>0</offset> <unit>V</unit> <defaultValue>0</defaultValue>\n        </Parameter>\n        <Parameter>\n          <name>Param 31</name> <direction>outgoing</direction> <encoding>BNR</encoding> <signed>true</signed> <startBit>1984 </startBit> <numberOfBits>64</numberOfBits> <scale>1</scale> <offset>0</offset> <unit>V</unit> <defaultValue>0</defaultValue>\n        </Parameter>\n        <Parameter>\n          <name>Param 32</name> <direction>outgoing</direction> <encoding>BNR</encoding> <signed>true</signed> <startBit>2048 </startBit> <numberOfBits>64</numberOfBits> <scale>1</scale> <offset>0</offset> <unit>V</unit> <defaultValue>0</defaultValue>\n        </Parameter>\n        <Parameter>\n          <name>Param 33</name> <direction>outgoing</direction> <encoding>BNR</encoding> <signed>true</signed> <startBit>2112 </startBit> <numberOfBits>64</numberOfBits> <scale>1</scale> <offset>0</offset> <unit>V</unit> <defaultValue>0</defaultValue>\n        </Parameter>\n        <Parameter>\n          <name>Param 34</name> <direction>outgoing</direction> <encoding>BNR</encoding> <signed>true</signed> <startBit>2176 </startBit> <numberOfBits>64</numberOfBits> <scale>1</scale> <offset>0</offset> <unit>V</unit> <defaultValue>0</defaultValue>\n        </Parameter>\n        <Parameter>\n          <name>Param 35</name> <direction>outgoing</direction> <encoding>BNR</encoding> <signed>true</signed> <startBit>2240 </startBit> <numberOfBits>64</numberOfBits> <scale>1</scale> <offset>0</offset> <unit>V</unit> <defaultValue>0</defaultValue>\n        </Parameter>\n        <Parameter>\n          <name>Param 36</name> <direction>outgoing</direction> <encoding>BNR</encoding> <signed>true</signed> <startBit>2304 </startBit> <numberOfBits>64</numberOfBits> <scale>1</scale> <offset>0</offset> <unit>V</unit> <defaultValue>0</defaultValue>\n        </Parameter>\n        <Parameter>\n          <name>Param 37</name> <direction>outgoing</direction> <encoding>BNR</encoding> <signed>true</signed> <startBit>2368 </startBit> <numberOfBits>64</numberOfBits> <scale>1</scale> <offset>0</offset> <unit>V</unit> <defaultValue>0</defaultValue>\n        </Parameter>\n        <Parameter>\n          <name>Param 38</name> <direction>outgoing</direction> <encoding>BNR</encoding> <signed>true</signed> <startBit>2432 </startBit> <numberOfBits>64</numberOfBits> <scale>1</scale> <offset>0</offset> <unit>V</unit> <defaultValue>0</defaultValue>\n        </Parameter>\n        <Parameter>\n          <name>Param 39</name> <direction>outgoing</direction> <encoding>BNR</encoding> <signed>true</signed> <startBit>2496 </startBit> <numberOfBits>64</numberOfBits> <scale>1</scale> <offset>0</offset> <unit>V</unit> <defaultValue>0</defaultValue>\n        </Parameter>\n        <Parameter>\n          <name>Param 40</name> <direction>outgoing</direction> <encoding>BNR</encoding> <signed>true</signed> <startBit>2560 </startBit> <numberOfBits>64</numberOfBits> <scale>1</scale> <offset>0</offset> <unit>V</unit> <defaultValue>0</defaultValue>\n        </Parameter>\n        <Parameter>\n          <name>Param 41</name> <direction>outgoing</direction> <encoding>BNR</encoding> <signed>true</signed> <startBit>2624 </startBit> <numberOfBits>64</numberOfBits> <scale>1</scale> <offset>0</offset> <unit>V</unit> <defaultValue>0</defaultValue>\n        </Parameter>\n        <Parameter>\n          <name>Param 42</name> <direction>outgoing</direction> <encoding>BNR</encoding> <signed>true</signed> <startBit>2688 </startBit> <numberOfBits>64</numberOfBits> <scale>1</scale> <offset>0</offset> <unit>V</unit> <defaultValue>0</defaultValue>\n        </Parameter>\n        <Parameter>\n          <name>Param 43</name> <direction>outgoing</direction> <encoding>BNR</encoding> <signed>true</signed> <startBit>2752 </startBit> <numberOfBits>64</numberOfBits> <scale>1</scale> <offset>0</offset> <unit>V</unit> <defaultValue>0</defaultValue>\n        </Parameter>\n        <Parameter>\n          <name>Param 44</name> <direction>outgoing</direction> <encoding>BNR</encoding> <signed>true</signed> <startBit>2816 </startBit> <numberOfBits>64</numberOfBits> <scale>1</scale> <offset>0</offset> <unit>V</unit> <defaultValue>0</defaultValue>\n        </Parameter>\n        <Parameter>\n          <name>Param 45</name> <direction>outgoing</direction> <encoding>BNR</encoding> <signed>true</signed> <startBit>2880 </startBit> <numberOfBits>64</numberOfBits> <scale>1</scale> <offset>0</offset> <unit>V</unit> <defaultValue>0</defaultValue>\n        </Parameter>\n        <Parameter>\n          <name>Param 46</name> <direction>outgoing</direction> <encoding>BNR</encoding> <signed>true</signed> <startBit>2944 </startBit> <numberOfBits>64</numberOfBits> <scale>1</scale> <offset>0</offset> <unit>V</unit> <defaultValue>0</defaultValue>\n        </Parameter>\n        <Parameter>\n          <name>Param 47</name> <direction>outgoing</direction> <encoding>BNR</encoding> <signed>true</signed> <startBit>3008 </startBit> <numberOfBits>64</numberOfBits> <scale>1</scale> <offset>0</offset> <unit>V</unit> <defaultValue>0</defaultValue>\n        </Parameter>\n        <Parameter>\n          <name>Param 48</name> <direction>outgoing</direction> <encoding>BNR</encoding> <signed>true</signed> <startBit>3072 </startBit> <numberOfBits>64</numberOfBits> <scale>1</scale> <offset>0</offset> <unit>V</unit> <defaultValue>0</defaultValue>\n        </Parameter>\n        <Parameter>\n          <name>Param 49</name> <direction>outgoing</direction> <encoding>BNR</encoding> <signed>true</signed> <startBit>3136 </startBit> <numberOfBits>64</numberOfBits> <scale>1</scale> <offset>0</offset> <unit>V</unit> <defaultValue>0</defaultValue>\n        </Parameter>\n        <Parameter>\n          <name>Param 50</name> <direction>outgoing</direction> <encoding>BNR</encoding> <signed>true</signed> <startBit>3200 </startBit> <numberOfBits>64</numberOfBits> <scale>1</scale> <offset>0</offset> <unit>V</unit> <defaultValue>0</defaultValue>\n        </Parameter>\n        <Parameter>\n          <name>Param 51</name> <direction>outgoing</direction> <encoding>BNR</encoding> <signed>true</signed> <startBit>3264 </startBit> <numberOfBits>64</numberOfBits> <scale>1</scale> <offset>0</offset> <unit>V</unit> <defaultValue>0</defaultValue>\n        </Parameter>\n        <Parameter>\n          <name>Param 52</name> <direction>outgoing</direction> <encoding>BNR</encoding> <signed>true</signed> <startBit>3328 </startBit> <numberOfBits>64</numberOfBits> <scale>1</scale> <offset>0</offset> <unit>V</unit> <defaultValue>0</defaultValue>\n        </Parameter>\n        <Parameter>\n          <name>Param 53</name> <direction>outgoing</direction> <encoding>BNR</encoding> <signed>true</signed> <startBit>3392 </startBit> <numberOfBits>64</numberOfBits> <scale>1</scale> <offset>0</offset> <unit>V</unit> <defaultValue>0</defaultValue>\n        </Parameter>\n        <Parameter>\n          <name>Param 54</name> <direction>outgoing</direction> <encoding>BNR</encoding> <signed>true</signed> <startBit>3456 </startBit> <numberOfBits>64</numberOfBits> <scale>1</scale> <offset>0</offset> <unit>V</unit> <defaultValue>0</defaultValue>\n        </Parameter>\n        <Parameter>\n          <name>Param 55</name> <direction>outgoing</direction> <encoding>BNR</encoding> <signed>true</signed> <startBit>3520 </startBit> <numberOfBits>64</numberOfBits> <scale>1</scale> <offset>0</offset> <unit>V</unit> <defaultValue>0</defaultValue>\n        </Parameter>\n        <Parameter>\n          <name>Param 56</name> <direction>outgoing</direction> <encoding>BNR</encoding> <signed>true</signed> <startBit>3584 </startBit> <numberOfBits>64</numberOfBits> <scale>1</scale> <offset>0</offset> <unit>V</unit> <defaultValue>0</defaultValue>\n        </Parameter>\n        <Parameter>\n          <name>Param 57</name> <direction>outgoing</direction> <encoding>BNR</encoding> <signed>true</signed> <startBit>3648 </startBit> <numberOfBits>64</numberOfBits> <scale>1</scale> <offset>0</offset> <unit>V</unit> <defaultValue>0</defaultValue>\n        </Parameter>\n        <Parameter>\n          <name>Param 58</name> <direction>outgoing</direction> <encoding>BNR</encoding> <signed>true</signed> <startBit>3712 </startBit> <numberOfBits>64</numberOfBits> <scale>1</scale> <offset>0</offset> <unit>V</unit> <defaultValue>0</defaultValue>\n        </Parameter>\n        <Parameter>\n          <name>Param 59</name> <direction>outgoing</direction> <encoding>BNR</encoding> <signed>true</signed> <startBit>3776 </startBit> <numberOfBits>64</numberOfBits> <scale>1</scale> <offset>0</offset> <unit>V</unit> <defaultValue>0</defaultValue>\n        </Parameter>\n        <Parameter>\n          <name>Param 60</name> <direction>outgoing</direction> <encoding>BNR</encoding> <signed>true</signed> <startBit>3840 </startBit> <numberOfBits>64</numberOfBits> <scale>1</scale> <offset>0</offset> <unit>V</unit> <defaultValue>0</defaultValue>\n        </Parameter>\n        <Parameter>\n          <name>Param 61</name> <direction>outgoing</direction> <encoding>BNR</encoding> <signed>true</signed> <startBit>3904 </startBit> <numberOfBits>64</numberOfBits> <scale>1</scale> <offset>0</offset> <unit>V</unit> <defaultValue>0</defaultValue>\n        </Parameter>\n        <Parameter>\n          <name>Param 62</name> <direction>outgoing</direction> <encoding>BNR</encoding> <signed>true</signed> <startBit>3968 </startBit> <numberOfBits>64</numberOfBits> <scale>1</scale> <offset>0</offset> <unit>V</unit> <defaultValue>0</defaultValue>\n        </Parameter>\n        <Parameter>\n          <name>Param 63</name> <direction>outgoing</direction> <encoding>BNR</encoding> <signed>true</signed> <startBit>4032 </startBit> <numberOfBits>64</numberOfBits> <scale>1</scale> <offset>0</offset> <unit>V</unit> <defaultValue>0</defaultValue>\n        </Parameter>\n        <Parameter>\n          <name>Param 64</name> <direction>outgoing</direction> <encoding>BNR</encoding> <signed>true</signed> <startBit>4096 </startBit> <numberOfBits>64</numberOfBits> <scale>1</scale> <offset>0</offset> <unit>V</unit> <defaultValue>0</defaultValue>\n        </Parameter>\n        <Parameter>\n          <name>Param 65</name> <direction>outgoing</direction> <encoding>BNR</encoding> <signed>true</signed> <startBit>4160 </startBit> <numberOfBits>64</numberOfBits> <scale>1</scale> <offset>0</offset> <unit>V</unit> <defaultValue>0</defaultValue>\n        </Parameter>\n        <Parameter>\n          <name>Param 66</name> <direction>outgoing</direction> <encoding>BNR</encoding> <signed>true</signed> <startBit>4224 </startBit> <numberOfBits>64</numberOfBits> <scale>1</scale> <offset>0</offset> <unit>V</unit> <defaultValue>0</defaultValue>\n        </Parameter>\n        <Parameter>\n          <name>Param 67</name> <direction>outgoing</direction> <encoding>BNR</encoding> <signed>true</signed> <startBit>4288 </startBit> <numberOfBits>64</numberOfBits> <scale>1</scale> <offset>0</offset> <unit>V</unit> <defaultValue>0</defaultValue>\n        </Parameter>\n        <Parameter>\n          <name>Param 68</name> <direction>outgoing</direction> <encoding>BNR</encoding> <signed>true</signed> <startBit>4352 </startBit> <numberOfBits>64</numberOfBits> <scale>1</scale> <offset>0</offset> <unit>V</unit> <defaultValue>0</defaultValue>\n        </Parameter>\n        <Parameter>\n          <name>Param 69</name> <direction>outgoing</direction> <encoding>BNR</encoding> <signed>true</signed> <startBit>4416 </startBit> <numberOfBits>64</numberOfBits> <scale>1</scale> <offset>0</offset> <unit>V</unit> <defaultValue>0</defaultValue>\n        </Parameter>\n        <Parameter>\n          <name>Param 70</name> <direction>outgoing</direction> <encoding>BNR</encoding> <signed>true</signed> <startBit>4480 </startBit> <numberOfBits>64</numberOfBits> <scale>1</scale> <offset>0</offset> <unit>V</unit> <defaultValue>0</defaultValue>\n        </Parameter>\n        <Parameter>\n          <name>Param 71</name> <direction>outgoing</direction> <encoding>BNR</encoding> <signed>true</signed> <startBit>4544 </startBit> <numberOfBits>64</numberOfBits> <scale>1</scale> <offset>0</offset> <unit>V</unit> <defaultValue>0</defaultValue>\n        </Parameter>\n        <Parameter>\n          <name>Param 72</name> <direction>outgoing</direction> <encoding>BNR</encoding> <signed>true</signed> <startBit>4608 </startBit> <numberOfBits>64</numberOfBits> <scale>1</scale> <offset>0</offset> <unit>V</unit> <defaultValue>0</defaultValue>\n        </Parameter>\n        <Parameter>\n          <name>Param 73</name> <direction>outgoing</direction> <encoding>BNR</encoding> <signed>true</signed> <startBit>4672 </startBit> <numberOfBits>64</numberOfBits> <scale>1</scale> <offset>0</offset> <unit>V</unit> <defaultValue>0</defaultValue>\n        </Parameter>\n        <Parameter>\n          <name>Param 74</name> <direction>outgoing</direction> <encoding>BNR</encoding> <signed>true</signed> <startBit>4736 </startBit> <numberOfBits>64</numberOfBits> <scale>1</scale> <offset>0</offset> <unit>V</unit> <defaultValue>0</defaultValue>\n        </Parameter>\n        <Parameter>\n          <name>Param 75</name> <direction>outgoing</direction> <encoding>BNR</encoding> <signed>true</signed> <startBit>4800 </startBit> <numberOfBits>64</numberOfBits> <scale>1</scale> <offset>0</offset> <unit>V</unit> <defaultValue>0</defaultValue>\n        </Parameter>\n        <Parameter>\n          <name>Param 76</name> <direction>outgoing</direction> <encoding>BNR</encoding> <signed>true</signed> <startBit>4864 </startBit> <numberOfBits>64</numberOfBits> <scale>1</scale> <offset>0</offset> <unit>V</unit> <defaultValue>0</defaultValue>\n        </Parameter>\n        <Parameter>\n          <name>Param 77</name> <direction>outgoing</direction> <encoding>BNR</encoding> <signed>true</signed> <startBit>4928 </startBit> <numberOfBits>64</numberOfBits> <scale>1</scale> <offset>0</offset> <unit>V</unit> <defaultValue>0</defaultValue>\n        </Parameter>\n        <Parameter>\n          <name>Param 78</name> <direction>outgoing</direction> <encoding>BNR</encoding> <signed>true</signed> <startBit>4992 </startBit> <numberOfBits>64</numberOfBits> <scale>1</scale> <offset>0</offset> <unit>V</unit> <defaultValue>0</defaultValue>\n        </Parameter>\n        <Parameter>\n          <name>Param 79</name> <direction>outgoing</direction> <encoding>BNR</encoding> <signed>true</signed> <startBit>5056 </startBit> <numberOfBits>64</numberOfBits> <scale>1</scale> <offset>0</offset> <unit>V</unit> <defaultValue>0</defaultValue>\n        </Parameter>\n        <Parameter>\n          <name>Param 80</name> <direction>outgoing</direction> <encoding>BNR</encoding> <signed>true</signed> <startBit>5120 </startBit> <numberOfBits>64</numberOfBits> <scale>1</scale> <offset>0</offset> <unit>V</unit> <defaultValue>0</defaultValue>\n        </Parameter>\n        <Parameter>\n          <name>Param 81</name> <direction>outgoing</direction> <encoding>BNR</encoding> <signed>true</signed> <startBit>5184 </startBit> <numberOfBits>64</numberOfBits> <scale>1</scale> <offset>0</offset> <unit>V</unit> <defaultValue>0</defaultValue>\n        </Parameter>\n        <Parameter>\n          <name>Param 82</name> <direction>outgoing</direction> <encoding>BNR</encoding> <signed>true</signed> <startBit>5248 </startBit> <numberOfBits>64</numberOfBits> <scale>1</scale> <offset>0</offset> <unit>V</unit> <defaultValue>0</defaultValue>\n        </Parameter>\n        <Parameter>\n          <name>Param 83</name> <direction>outgoing</direction> <encoding>BNR</encoding> <signed>true</signed> <startBit>5312 </startBit> <numberOfBits>64</numberOfBits> <scale>1</scale> <offset>0</offset> <unit>V</unit> <defaultValue>0</defaultValue>\n        </Parameter>\n        <Parameter>\n          <name>Param 84</name> <direction>outgoing</direction> <encoding>BNR</encoding> <signed>true</signed> <startBit>5376 </startBit> <numberOfBits>64</numberOfBits> <scale>1</scale> <offset>0</offset> <unit>V</unit> <defaultValue>0</defaultValue>\n        </Parameter>\n        <Parameter>\n          <name>Param 85</name> <direction>outgoing</direction> <encoding>BNR</encoding> <signed>true</signed> <startBit>5440 </startBit> <numberOfBits>64</numberOfBits> <scale>1</scale> <offset>0</offset> <unit>V</unit> <defaultValue>0</defaultValue>\n        </Parameter>\n        <Parameter>\n          <name>Param 86</name> <direction>outgoing</direction> <encoding>BNR</encoding> <signed>true</signed> <startBit>5504 </startBit> <numberOfBits>64</numberOfBits> <scale>1</scale> <offset>0</offset> <unit>V</unit> <defaultValue>0</defaultValue>\n        </Parameter>\n        <Parameter>\n          <name>Param 87</name> <direction>outgoing</direction> <encoding>BNR</encoding> <signed>true</signed> <startBit>5568 </startBit> <numberOfBits>64</numberOfBits> <scale>1</scale> <offset>0</offset> <unit>V</unit> <defaultValue>0</defaultValue>\n        </Parameter>\n        <Parameter>\n          <name>Param 88</name> <direction>outgoing</direction> <encoding>BNR</encoding> <signed>true</signed> <startBit>5632 </startBit> <numberOfBits>64</numberOfBits> <scale>1</scale> <offset>0</offset> <unit>V</unit> <defaultValue>0</defaultValue>\n        </Parameter>\n        <Parameter>\n          <name>Param 89</name> <direction>outgoing</direction> <encoding>BNR</encoding> <signed>true</signed> <startBit>5696 </startBit> <numberOfBits>64</numberOfBits> <scale>1</scale> <offset>0</offset> <unit>V</unit> <defaultValue>0</defaultValue>\n        </Parameter>\n        <Parameter>\n          <name>Param 90</name> <direction>outgoing</direction> <encoding>BNR</encoding> <signed>true</signed> <startBit>5760 </startBit> <numberOfBits>64</numberOfBits> <scale>1</scale> <offset>0</offset> <unit>V</unit> <defaultValue>0</defaultValue>\n        </Parameter>\n        <Parameter>\n          <name>Param 91</name> <direction>outgoing</direction> <encoding>BNR</encoding> <signed>true</signed> <startBit>5824 </startBit> <numberOfBits>64</numberOfBits> <scale>1</scale> <offset>0</offset> <unit>V</unit> <defaultValue>0</defaultValue>\n        </Parameter>\n        <Parameter>\n          <name>Param 92</name> <direction>outgoing</direction> <encoding>BNR</encoding> <signed>true</signed> <startBit>5888 </startBit> <numberOfBits>64</numberOfBits> <scale>1</scale> <offset>0</offset> <unit>V</unit> <defaultValue>0</defaultValue>\n        </Parameter>\n        <Parameter>\n          <name>Param 93</name> <direction>outgoing</direction> <encoding>BNR</encoding> <signed>true</signed> <startBit>5952 </startBit> <numberOfBits>64</numberOfBits> <scale>1</scale> <offset>0</offset> <unit>V</unit> <defaultValue>0</defaultValue>\n        </Parameter>\n        <Parameter>\n          <name>Param 94</name> <direction>outgoing</direction> <encoding>BNR</encoding> <signed>true</signed> <startBit>6016 </startBit> <numberOfBits>64</numberOfBits> <scale>1</scale> <offset>0</offset> <unit>V</unit> <defaultValue>0</defaultValue>\n        </Parameter>\n        <Parameter>\n          <name>Param 95</name> <direction>outgoing</direction> <encoding>BNR</encoding> <signed>true</signed> <startBit>6080 </startBit> <numberOfBits>64</numberOfBits> <scale>1</scale> <offset>0</offset> <unit>V</unit> <defaultValue>0</defaultValue>\n        </Parameter>\n        <Parameter>\n          <name>Param 96</name> <direction>outgoing</direction> <encoding>BNR</encoding> <signed>true</signed> <startBit>6144 </startBit> <numberOfBits>64</numberOfBits> <scale>1</scale> <offset>0</offset> <unit>V</unit> <defaultValue>0</defaultValue>\n        </Parameter>\n        <Parameter>\n          <name>Param 97</name> <direction>outgoing</direction> <encoding>BNR</encoding> <signed>true</signed> <startBit>6208 </startBit> <numberOfBits>64</numberOfBits> <scale>1</scale> <offset>0</offset> <unit>V</unit> <defaultValue>0</defaultValue>\n        </Parameter>\n        <Parameter>\n          <name>Param 98</name> <direction>outgoing</direction> <encoding>BNR</encoding> <signed>true</signed> <startBit>6272 </startBit> <numberOfBits>64</numberOfBits> <scale>1</scale> <offset>0</offset> <unit>V</unit> <defaultValue>0</defaultValue>\n        </Parameter>\n        <Parameter>\n          <name>Param 99</name> <direction>outgoing</direction> <encoding>BNR</encoding> <signed>true</signed> <startBit>6336 </startBit> <numberOfBits>64</numberOfBits> <scale>1</scale> <offset>0</offset> <unit>V</unit> <defaultValue>0</defaultValue>\n        </Parameter>\n        <Parameter>\n          <name>Param 100</name> <direction>outgoing</direction> <encoding>BNR</encoding> <signed>true</signed> <startBit>6400 </startBit> <numberOfBits>64</numberOfBits> <scale>1</scale> <offset>0</offset> <unit>V</unit> <defaultValue>0</defaultValue>\n        </Parameter>\n        <Parameter>\n          <name>Param 101</name> <direction>outgoing</direction> <encoding>BNR</encoding> <signed>true</signed> <startBit>6464 </startBit> <numberOfBits>64</numberOfBits> <scale>1</scale> <offset>0</offset> <unit>V</unit> <defaultValue>0</defaultValue>\n        </Parameter>\n        <Parameter>\n          <name>Param 102</name> <direction>outgoing</direction> <encoding>BNR</encoding> <signed>true</signed> <startBit>6528 </startBit> <numberOfBits>64</numberOfBits> <scale>1</scale> <offset>0</offset> <unit>V</unit> <defaultValue>0</defaultValue>\n        </Parameter>\n        <Parameter>\n          <name>Param 103</name> <direction>outgoing</direction> <encoding>BNR</encoding> <signed>true</signed> <startBit>6592 </startBit> <numberOfBits>64</numberOfBits> <scale>1</scale> <offset>0</offset> <unit>V</unit> <defaultValue>0</defaultValue>\n        </Parameter>\n        <Parameter>\n          <name>Param 104</name> <direction>outgoing</direction> <encoding>BNR</encoding> <signed>true</signed> <startBit>6656 </startBit> <numberOfBits>64</numberOfBits> <scale>1</scale> <offset>0</offset> <unit>V</unit> <defaultValue>0</defaultValue>\n        </Parameter>\n        <Parameter>\n          <name>Param 105</name> <direction>outgoing</direction> <encoding>BNR</encoding> <signed>true</signed> <startBit>6720 </startBit> <numberOfBits>64</numberOfBits> <scale>1</scale> <offset>0</offset> <unit>V</unit> <defaultValue>0</defaultValue>\n        </Parameter>\n        <Parameter>\n          <name>Param 106</name> <direction>outgoing</direction> <encoding>BNR</encoding> <signed>true</signed> <startBit>6784 </startBit> <numberOfBits>64</numberOfBits> <scale>1</scale> <offset>0</offset> <unit>V</unit> <defaultValue>0</defaultValue>\n        </Parameter>\n        <Parameter>\n          <name>Param 107</name> <direction>outgoing</direction> <encoding>BNR</encoding> <signed>true</signed> <startBit>6848 </startBit> <numberOfBits>64</numberOfBits> <scale>1</scale> <offset>0</offset> <unit>V</unit> <defaultValue>0</defaultValue>\n        </Parameter>\n        <Parameter>\n          <name>Param 108</name> <direction>outgoing</direction> <encoding>BNR</encoding> <signed>true</signed> <startBit>6912 </startBit> <numberOfBits>64</numberOfBits> <scale>1</scale> <offset>0</offset> <unit>V</unit> <defaultValue>0</defaultValue>\n        </Parameter>\n        <Parameter>\n          <name>Param 109</name> <direction>outgoing</direction> <encoding>BNR</encoding> <signed>true</signed> <startBit>6976 </startBit> <numberOfBits>64</numberOfBits> <scale>1</scale> <offset>0</offset> <unit>V</unit> <defaultValue>0</defaultValue>\n        </Parameter>\n        <Parameter>\n          <name>Param 110</name> <direction>outgoing</direction> <encoding>BNR</encoding> <signed>true</signed> <startBit>7040 </startBit> <numberOfBits>64</numberOfBits> <scale>1</scale> <offset>0</offset> <unit>V</unit> <defaultValue>0</defaultValue>\n        </Parameter>\n        <Parameter>\n          <name>Param 111</name> <direction>outgoing</direction> <encoding>BNR</encoding> <signed>true</signed> <startBit>7104 </startBit> <numberOfBits>64</numberOfBits> <scale>1</scale> <offset>0</offset> <unit>V</unit> <defaultValue>0</defaultValue>\n        </Parameter>\n        <Parameter>\n          <name>Param 112</name> <direction>outgoing</direction> <encoding>BNR</encoding> <signed>true</signed> <startBit>7168 </startBit> <numberOfBits>64</numberOfBits> <scale>1</scale> <offset>0</offset> <unit>V</unit> <defaultValue>0</defaultValue>\n        </Parameter>\n        <Parameter>\n          <name>Param 113</name> <direction>outgoing</direction> <encoding>BNR</encoding> <signed>true</signed> <startBit>7232 </startBit> <numberOfBits>64</numberOfBits> <scale>1</scale> <offset>0</offset> <unit>V</unit> <defaultValue>0</defaultValue>\n        </Parameter>\n        <Parameter>\n          <name>Param 114</name> <direction>outgoing</direction> <encoding>BNR</encoding> <signed>true</signed> <startBit>7296 </startBit> <numberOfBits>64</numberOfBits> <scale>1</scale> <offset>0</offset> <unit>V</unit> <defaultValue>0</defaultValue>\n        </Parameter>\n        <Parameter>\n          <name>Param 115</name> <direction>outgoing</direction> <encoding>BNR</encoding> <signed>true</signed> <startBit>7360 </startBit> <numberOfBits>64</numberOfBits> <scale>1</scale> <offset>0</offset> <unit>V</unit> <defaultValue>0</defaultValue>\n        </Parameter>\n        <Parameter>\n          <name>Param 116</name> <direction>outgoing</direction> <encoding>BNR</encoding> <signed>true</signed> <startBit>7424 </startBit> <numberOfBits>64</numberOfBits> <scale>1</scale> <offset>0</offset> <unit>V</unit> <defaultValue>0</defaultValue>\n        </Parameter>\n        <Parameter>\n          <name>Param 117</name> <direction>outgoing</direction> <encoding>BNR</encoding> <signed>true</signed> <startBit>7488 </startBit> <numberOfBits>64</numberOfBits> <scale>1</scale> <offset>0</offset> <unit>V</unit> <defaultValue>0</defaultValue>\n        </Parameter>\n        <Parameter>\n          <name>Param 118</name> <direction>outgoing</direction> <encoding>BNR</encoding> <signed>true</signed> <startBit>7552 </startBit> <numberOfBits>64</numberOfBits> <scale>1</scale> <offset>0</offset> <unit>V</unit> <defaultValue>0</defaultValue>\n        </Parameter>\n        <Parameter>\n          <name>Param 119</name> <direction>outgoing</direction> <encoding>BNR</encoding> <signed>true</signed> <startBit>7616 </startBit> <numberOfBits>64</numberOfBits> <scale>1</scale> <offset>0</offset> <unit>V</unit> <defaultValue>0</defaultValue>\n        </Parameter>\n        <Parameter>\n          <name>Param 120</name> <direction>outgoing</direction> <encoding>BNR</encoding> <signed>true</signed> <startBit>7680 </startBit> <numberOfBits>64</numberOfBits> <scale>1</scale> <offset>0</offset> <unit>V</unit> <defaultValue>0</defaultValue>\n        </Parameter>\n        <Parameter>\n          <name>Param 121</name> <direction>outgoing</direction> <encoding>BNR</encoding> <signed>true</signed> <startBit>7744 </startBit> <numberOfBits>64</numberOfBits> <scale>1</scale> <offset>0</offset> <unit>V</unit> <defaultValue>0</defaultValue>\n        </Parameter>\n        <Parameter>\n          <name>Param 122</name> <direction>outgoing</direction> <encoding>BNR</encoding> <signed>true</signed> <startBit>7808 </startBit> <numberOfBits>64</numberOfBits> <scale>1</scale> <offset>0</offset> <unit>V</unit> <defaultValue>0</defaultValue>\n        </Parameter>\n        <Parameter>\n          <name>Param 123</name> <direction>outgoing</direction> <encoding>BNR</encoding> <signed>true</signed> <startBit>7872 </startBit> <numberOfBits>64</numberOfBits> <scale>1</scale> <offset>0</offset> <unit>V</unit> <defaultValue>0</defaultValue>\n        </Parameter>\n        <Parameter>\n          <name>Param 124</name> <direction>outgoing</direction> <encoding>BNR</encoding> <signed>true</signed> <startBit>7936 </startBit> <numberOfBits>64</numberOfBits> <scale>1</scale> <offset>0</offset> <unit>V</unit> <defaultValue>0</defaultValue>\n        </Parameter>\n        <Parameter>\n          <name>Param 125</name> <direction>outgoing</direction> <encoding>BNR</encoding> <signed>true</signed> <startBit>8000 </startBit> <numberOfBits>64</numberOfBits> <scale>1</scale> <offset>0</offset> <unit>V</unit> <defaultValue>0</defaultValue>\n        </Parameter>\n        <Parameter>\n          <name>Param 126</name> <direction>outgoing</direction> <encoding>BNR</encoding> <signed>true</signed> <startBit>8064 </startBit> <numberOfBits>64</numberOfBits> <scale>1</scale> <offset>0</offset> <unit>V</unit> <defaultValue>0</defaultValue>\n        </Parameter>\n        <Parameter>\n          <name>Param 127</name> <direction>outgoing</direction> <encoding>BNR</encoding> <signed>true</signed> <startBit>8128 </startBit> <numberOfBits>64</numberOfBits> <scale>1</scale> <offset>0</offset> <unit>V</unit> <defaultValue>0</defaultValue>\n        </Parameter>\n        <Parameter>\n          <name>Param 128</name> <direction>outgoing</direction> <encoding>BNR</encoding> <signed>true</signed> <startBit>8192 </startBit> <numberOfBits>64</numberOfBits> <scale>1</scale> <offset>0</offset> <unit>V</unit> <defaultValue>0</defaultValue>\n        </Parameter>\n        <Parameter>\n          <name>Param 129</name> <direction>outgoing</direction> <encoding>BNR</encoding> <signed>true</signed> <startBit>8256 </startBit> <numberOfBits>64</numberOfBits> <scale>1</scale> <offset>0</offset> <unit>V</unit> <defaultValue>0</defaultValue>\n        </Parameter>\n        <Parameter>\n          <name>Param 130</name> <direction>outgoing</direction> <encoding>BNR</encoding> <signed>true</signed> <startBit>8320 </startBit> <numberOfBits>64</numberOfBits> <scale>1</scale> <offset>0</offset> <unit>V</unit> <defaultValue>0</defaultValue>\n        </Parameter>\n        <Parameter>\n          <name>Param 131</name> <direction>outgoing</direction> <encoding>BNR</encoding> <signed>true</signed> <startBit>8384 </startBit> <numberOfBits>64</numberOfBits> <scale>1</scale> <offset>0</offset> <unit>V</unit> <defaultValue>0</defaultValue>\n        </Parameter>\n        <Parameter>\n          <name>Param 132</name> <direction>outgoing</direction> <encoding>BNR</encoding> <signed>true</signed> <startBit>8448 </startBit> <numberOfBits>64</numberOfBits> <scale>1</scale> <offset>0</offset> <unit>V</unit> <defaultValue>0</defaultValue>\n        </Parameter>\n        <Parameter>\n          <name>Param 133</name> <direction>outgoing</direction> <encoding>BNR</encoding> <signed>true</signed> <startBit>8512 </startBit> <numberOfBits>64</numberOfBits> <scale>1</scale> <offset>0</offset> <unit>V</unit> <defaultValue>0</defaultValue>\n        </Parameter>\n        <Parameter>\n          <name>Param 134</name> <direction>outgoing</direction> <encoding>BNR</encoding> <signed>true</signed> <startBit>8576 </startBit> <numberOfBits>64</numberOfBits> <scale>1</scale> <offset>0</offset> <unit>V</unit> <defaultValue>0</defaultValue>\n        </Parameter>\n        <Parameter>\n          <name>Param 135</name> <direction>outgoing</direction> <encoding>BNR</encoding> <signed>true</signed> <startBit>8640 </startBit> <numberOfBits>64</numberOfBits> <scale>1</scale> <offset>0</offset> <unit>V</unit> <defaultValue>0</defaultValue>\n        </Parameter>\n        <Parameter>\n          <name>Param 136</name> <direction>outgoing</direction> <encoding>BNR</encoding> <signed>true</signed> <startBit>8704 </startBit> <numberOfBits>64</numberOfBits> <scale>1</scale> <offset>0</offset> <unit>V</unit> <defaultValue>0</defaultValue>\n        </Parameter>\n        <Parameter>\n          <name>Param 137</name> <direction>outgoing</direction> <encoding>BNR</encoding> <signed>true</signed> <startBit>8768 </startBit> <numberOfBits>64</numberOfBits> <scale>1</scale> <offset>0</offset> <unit>V</unit> <defaultValue>0</defaultValue>\n        </Parameter>\n        <Parameter>\n          <name>Param 138</name> <direction>outgoing</direction> <encoding>BNR</encoding> <signed>true</signed> <startBit>8832 </startBit> <numberOfBits>64</numberOfBits> <scale>1</scale> <offset>0</offset> <unit>V</unit> <defaultValue>0</defaultValue>\n        </Parameter>\n        <Parameter>\n          <name>Param 139</name> <direction>outgoing</direction> <encoding>BNR</encoding> <signed>true</signed> <startBit>8896 </startBit> <numberOfBits>64</numberOfBits> <scale>1</scale> <offset>0</offset> <unit>V</unit> <defaultValue>0</defaultValue>\n        </Parameter>\n        <Parameter>\n          <name>Param 140</name> <direction>outgoing</direction> <encoding>BNR</encoding> <signed>true</signed> <startBit>8960 </startBit> <numberOfBits>64</numberOfBits> <scale>1</scale> <offset>0</offset> <unit>V</unit> <defaultValue>0</defaultValue>\n        </Parameter>\n        <Parameter>\n          <name>Param 141</name> <direction>outgoing</direction> <encoding>BNR</encoding> <signed>true</signed> <startBit>9024 </startBit> <numberOfBits>64</numberOfBits> <scale>1</scale> <offset>0</offset> <unit>V</unit> <defaultValue>0</defaultValue>\n        </Parameter>\n        <Parameter>\n          <name>Param 142</name> <direction>outgoing</direction> <encoding>BNR</encoding> <signed>true</signed> <startBit>9088 </startBit> <numberOfBits>64</numberOfBits> <scale>1</scale> <offset>0</offset> <unit>V</unit> <defaultValue>0</defaultValue>\n        </Parameter>\n        <Parameter>\n          <name>Param 143</name> <direction>outgoing</direction> <encoding>BNR</encoding> <signed>true</signed> <startBit>9152 </startBit> <numberOfBits>64</numberOfBits> <scale>1</scale> <offset>0</offset> <unit>V</unit> <defaultValue>0</defaultValue>\n        </Parameter>\n        <Parameter>\n          <name>Param 144</name> <direction>outgoing</direction> <encoding>BNR</encoding> <signed>true</signed> <startBit>9216 </startBit> <numberOfBits>64</numberOfBits> <scale>1</scale> <offset>0</offset> <unit>V</unit> <defaultValue>0</defaultValue>\n        </Parameter>\n        <Parameter>\n          <name>Param 145</name> <direction>outgoing</direction> <encoding>BNR</encoding> <signed>true</signed> <startBit>9280 </startBit> <numberOfBits>64</numberOfBits> <scale>1</scale> <offset>0</offset> <unit>V</unit> <defaultValue>0</defaultValue>\n        </Parameter>\n        <Parameter>\n          <name>Param 146</name> <direction>outgoing</direction> <encoding>BNR</encoding> <signed>true</signed> <startBit>9344 </startBit> <numberOfBits>64</numberOfBits> <scale>1</scale> <offset>0</offset> <unit>V</unit> <defaultValue>0</defaultValue>\n        </Parameter>\n        <Parameter>\n          <name>Param 147</name> <direction>outgoing</direction> <encoding>BNR</encoding> <signed>true</signed> <startBit>9408 </startBit> <numberOfBits>64</numberOfBits> <scale>1</scale> <offset>0</offset> <unit>V</unit> <defaultValue>0</defaultValue>\n        </Parameter>\n        <Parameter>\n          <name>Param 148</name> <direction>outgoing</direction> <encoding>BNR</encoding> <signed>true</signed> <startBit>9472 </startBit> <numberOfBits>64</numberOfBits> <scale>1</scale> <offset>0</offset> <unit>V</unit> <defaultValue>0</defaultValue>\n        </Parameter>\n        <Parameter>\n          <name>Param 149</name> <direction>outgoing</direction> <encoding>BNR</encoding> <signed>true</signed> <startBit>9536 </startBit> <numberOfBits>64</numberOfBits> <scale>1</scale> <offset>0</offset> <unit>V</unit> <defaultValue>0</defaultValue>\n        </Parameter>\n        <Parameter>\n          <name>Param 150</name> <direction>outgoing</direction> <encoding>BNR</encoding> <signed>true</signed> <startBit>9600 </startBit> <numberOfBits>64</numberOfBits> <scale>1</scale> <offset>0</offset> <unit>V</unit> <defaultValue>0</defaultValue>\n        </Parameter>\n        <Parameter>\n          <name>Param 151</name> <direction>outgoing</direction> <encoding>BNR</encoding> <signed>true</signed> <startBit>9664 </startBit> <numberOfBits>64</numberOfBits> <scale>1</scale> <offset>0</offset> <unit>V</unit> <defaultValue>0</defaultValue>\n        </Parameter>\n        <Parameter>\n          <name>Param 152</name> <direction>outgoing</direction> <encoding>BNR</encoding> <signed>true</signed> <startBit>9728 </startBit> <numberOfBits>64</numberOfBits> <scale>1</scale> <offset>0</offset> <unit>V</unit> <defaultValue>0</defaultValue>\n        </Parameter>\n        <Parameter>\n          <name>Param 153</name> <direction>outgoing</direction> <encoding>BNR</encoding> <signed>true</signed> <startBit>9792 </startBit> <numberOfBits>64</numberOfBits> <scale>1</scale> <offset>0</offset> <unit>V</unit> <defaultValue>0</defaultValue>\n        </Parameter>\n        <Parameter>\n          <name>Param 154</name> <direction>outgoing</direction> <encoding>BNR</encoding> <signed>true</signed> <startBit>9856 </startBit> <numberOfBits>64</numberOfBits> <scale>1</scale> <offset>0</offset> <unit>V</unit> <defaultValue>0</defaultValue>\n        </Parameter>\n        <Parameter>\n          <name>Param 155</name> <direction>outgoing</direction> <encoding>BNR</encoding> <signed>true</signed> <startBit>9920 </startBit> <numberOfBits>64</numberOfBits> <scale>1</scale> <offset>0</offset> <unit>V</unit> <defaultValue>0</defaultValue>\n        </Parameter>\n        <Parameter>\n          <name>Param 156</name> <direction>outgoing</direction> <encoding>BNR</encoding> <signed>true</signed> <startBit>9984 </startBit> <numberOfBits>64</numberOfBits> <scale>1</scale> <offset>0</offset> <unit>V</unit> <defaultValue>0</defaultValue>\n        </Parameter>\n        <Parameter>\n          <name>Param 157</name> <direction>outgoing</direction> <encoding>BNR</encoding> <signed>true</signed> <startBit>10048 </startBit> <numberOfBits>64</numberOfBits> <scale>1</scale> <offset>0</offset> <unit>V</unit> <defaultValue>0</defaultValue>\n        </Parameter>\n        <Parameter>\n          <name>Param 158</name> <direction>outgoing</direction> <encoding>BNR</encoding> <signed>true</signed> <startBit>10112 </startBit> <numberOfBits>64</numberOfBits> <scale>1</scale> <offset>0</offset> <unit>V</unit> <defaultValue>0</defaultValue>\n        </Parameter>\n        <Parameter>\n          <name>Param 159</name> <direction>outgoing</direction> <encoding>BNR</encoding> <signed>true</signed> <startBit>10176 </startBit> <numberOfBits>64</numberOfBits> <scale>1</scale> <offset>0</offset> <unit>V</unit> <defaultValue>0</defaultValue>\n        </Parameter>\t   \n     </TxCommPort>\n    </TxUdpSession>\n  </Port>\n</Board>"
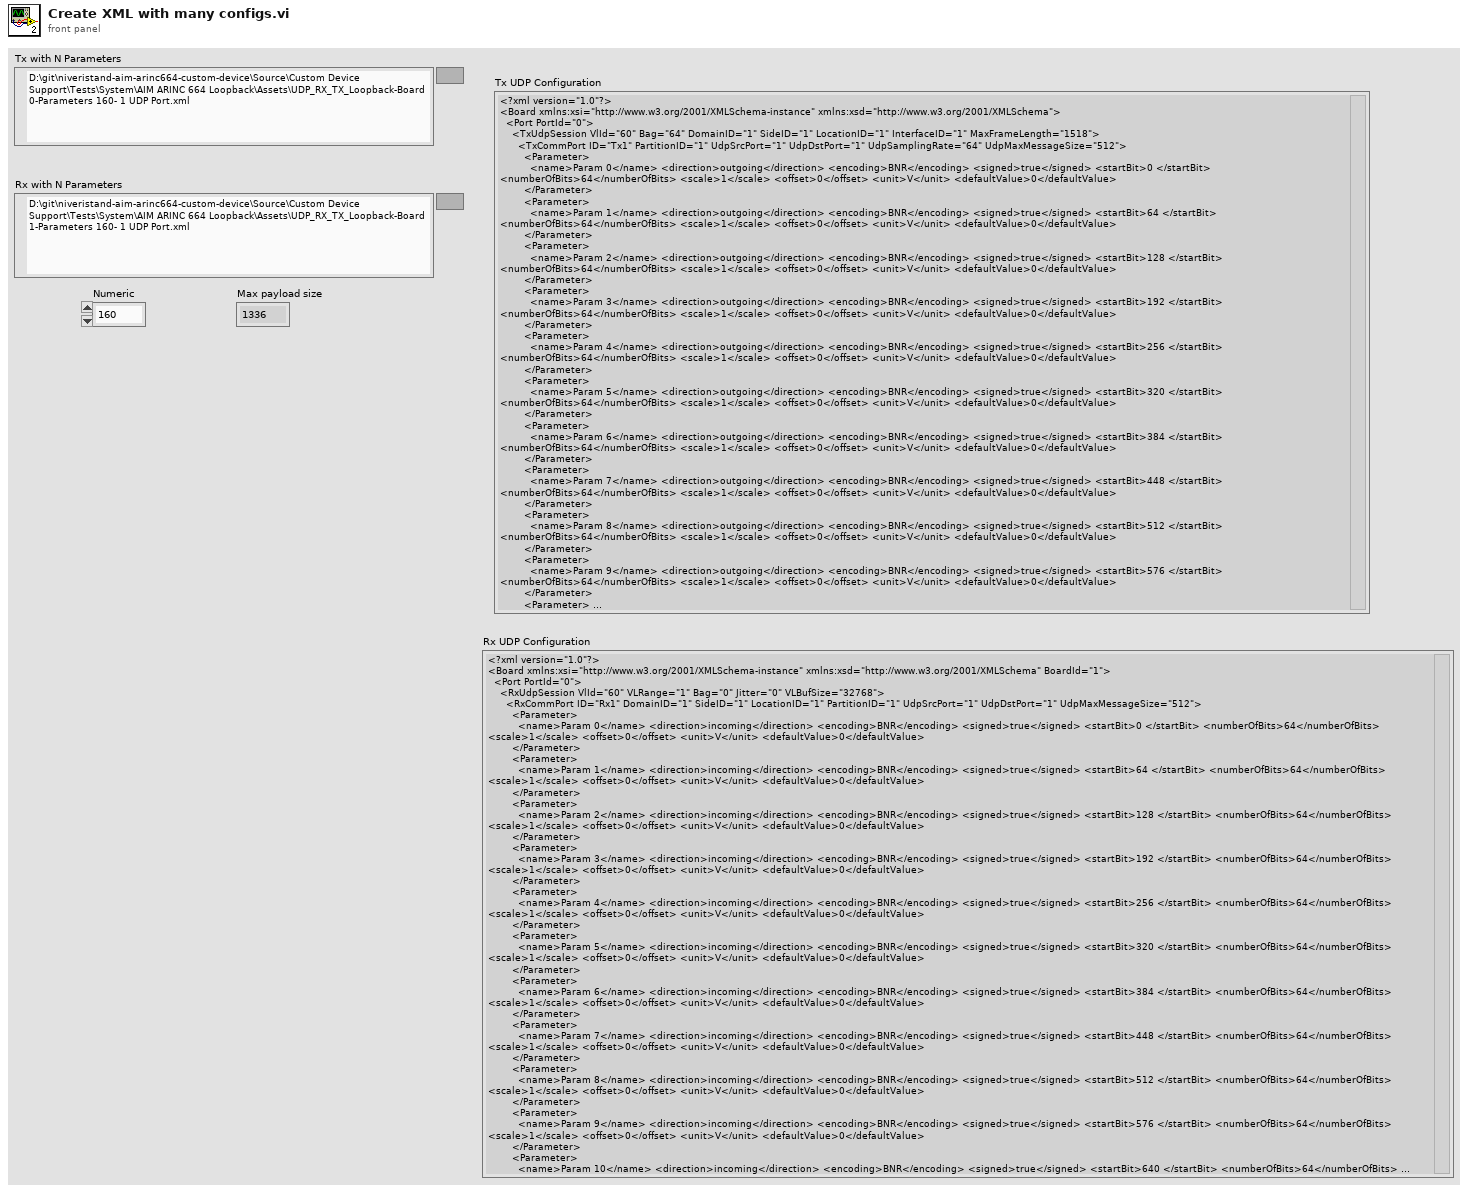
[diagram p1: front panel]
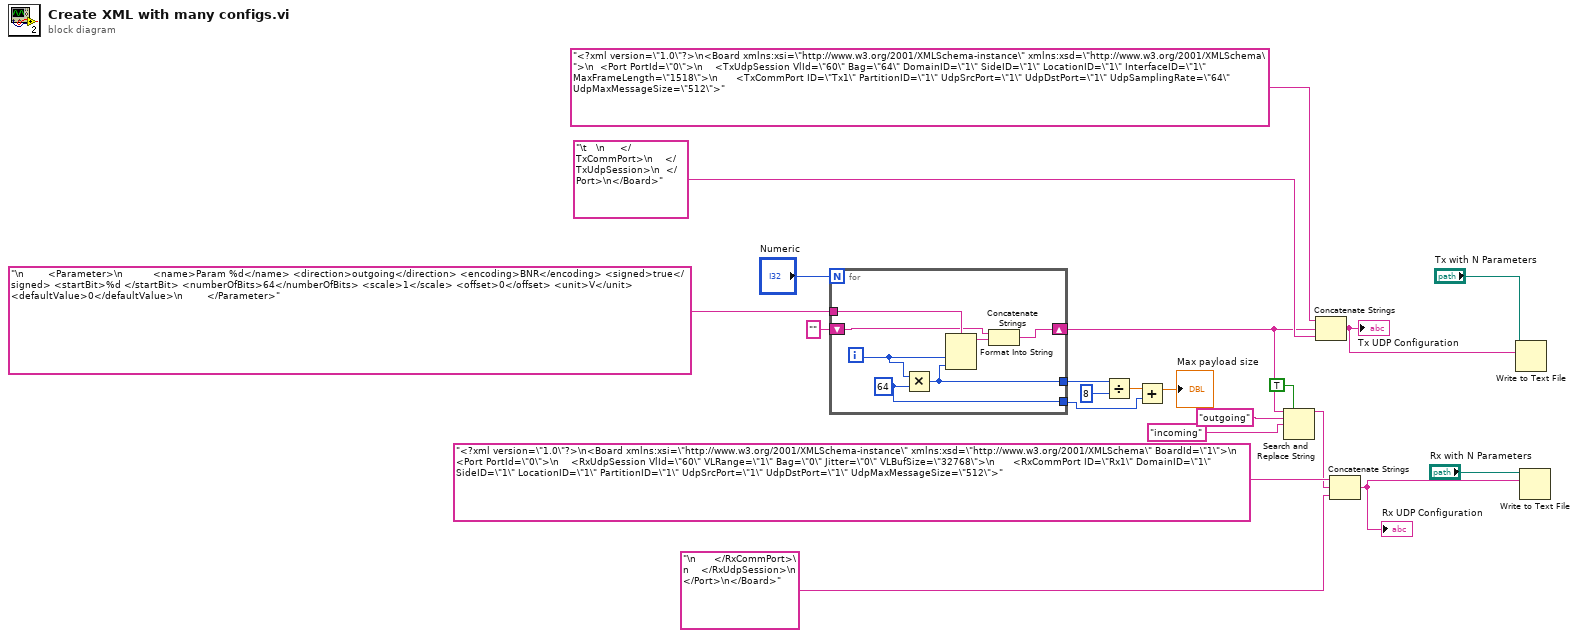
[diagram p0: block diagram]
diagram:
  n1 = for {
    N: "Numeric" -> [_]
    tunnel: "\n        <Parameter>\n          <name>Param %d</name> <direction>outgoing</direction> <encoding>BNR</encoding> <signed>true</signed> <startBit>%d </startBit> <numberOfBits>64</numberOfBits> <scale>1</scale> <offset>0</offset> <unit>V</unit> <defaultValue>0</defaultValue>\n        </Parameter>" -> [w28]
    shift-right: [w24] -> w5
    shift-left: "" -> [w25]
    tunnel: [w23] -> w10
    tunnel: [w22] -> w6
    i -> [w27]
    w22 = 64 ("y")
    n2 = Multiply(x=w27, y=w22) -> (x*y=w23:i32)
    n3 = Format Into String(format string=w28, w27, w23) -> (resulting string=w26:string)  [unwired: 2 in, 1 out]
    n4 = Concatenate Strings(w25, w26) -> (w24:string)
  }
  n5 = Divide(x=w10, y=8) -> (x/y=w8:dbl)
  n6 = Add(x=w8, y=w6) -> (x+y=→"Max payload size":dbl)
  n7 = Search and Replace String(replace all?=TRUE ("replace all? (F)"), input string=w5, search string="outgoing", replace string="incoming" ("replace string (\"\")")) -> (result string=w4:string)  [unwired: 4 in, 3 out]
  n8 = Concatenate Strings("<?xml version=\"1.0\"?>\n<Board xmlns:xsi=\"http://www.w3.org/2001/XMLSchema-instance\" xmlns:xsd=\"http://www.w3.org/2001/XMLSchema\">\n  <Port PortId=\"0\">\n    <TxUdpSession VlId=\"60\" Bag=\"64\" DomainID=\"1\" SideID=\"1\" LocationID=\"1\" InterfaceID=\"1\" MaxFrameLength=\"1518\">\n      <TxCommPort ID=\"Tx1\" PartitionID=\"1\" UdpSrcPort=\"1\" UdpDstPort=\"1\" UdpSamplingRate=\"64\" UdpMaxMessageSize=\"512\">", w5, "\t   \n     </TxCommPort>\n    </TxUdpSession>\n  </Port>\n</Board>") -> (w17:string)
  "Tx UDP Configuration" <- w17
  n9 = Concatenate Strings("<?xml version=\"1.0\"?>\n<Board xmlns:xsi=\"http://www.w3.org/2001/XMLSchema-instance\" xmlns:xsd=\"http://www.w3.org/2001/XMLSchema\" BoardId=\"1\">\n  <Port PortId=\"0\">\n    <RxUdpSession VlId=\"60\" VLRange=\"1\" Bag=\"0\" Jitter=\"0\" VLBufSize=\"32768\">\n      <RxCommPort ID=\"Rx1\" DomainID=\"1\" SideID=\"1\" LocationID=\"1\" PartitionID=\"1\" UdpSrcPort=\"1\" UdpDstPort=\"1\" UdpMaxMessageSize=\"512\">", w4, "\n      </RxCommPort>\n    </RxUdpSession>\n  </Port>\n</Board>") -> (w12:string)
  "Rx UDP Configuration" <- w12
  n10 = Write to Text File(file (use dialog)="Tx with N Parameters", text=w17) -> ()  [unwired: 2 in, 3 out]
  n11 = Write to Text File(file (use dialog)="Rx with N Parameters", text=w12) -> ()  [unwired: 2 in, 3 out]
